vi "Autopatch-v2_mp285.vi"() -> ()   [LabVIEW 2018]
uses:
  <vilib>/vision/driver/NI_Vision_Acquisition_Software.lvlib
  <vilib>/DAQmx/create/channels.llb/DAQmx Create Channel (AO-Voltage-Basic).vi
  <vilib>/DAQmx/configure/timing.llb/DAQmx Timing (Sample Clock).vi
  <resource>/objmgr/daqmx.rc
  <vilib>/Analysis/NI_AALBase.lvlib
  <vilib>/Analysis/baseanly.llb/Mean (DBL).vi
  <vilib>/measure/NI_MABase.lvlib
  <vilib>/vision/NI_Vision_Development_Module.lvlib
  <vilib>/addons/control/pid/NI_PID_pid.lvlib
  <vilib>/addons/control/pid/pid.llb/PID (DBL).vi
  <vilib>/Analysis/NI_AALPro.lvlib
  <vilib>/DAQmx/write.llb/DAQmx Write (Analog DBL 1Chan 1Samp).vi
  <vilib>/DAQmx/configure/trigger.llb/DAQmx Start Trigger (Digital Edge).vi
  <vilib>/Waveform/WDTOps.llb/WDT Waveform Duration DBL.vi
  <vilib>/DAQmx/read.llb/DAQmx Read (Analog Wfm 1Chan NSamp).vi
  <vilib>/DAQmx/create/channels.llb/DAQmx Create Channel (AI-Voltage-Basic).vi
  <vilib>/DAQmx/write.llb/DAQmx Write (Analog Wfm 1Chan NSamp).vi
  <vilib>/userdefined/High Color/IMAQdx.ctl
panel:
  out "数据输出 2":string
  in  "模式（标准） 2":T1(ring)
  out "写入的字节 2":i32
  out "元素":string
  in  "自动对焦状态机":u16(ring) items=["自动对焦初始", "自动对焦循环", "自动对焦结束"]
  in  "自动扫描状态机":u16(ring) items=["自动扫描初始", "自动扫描循环", "自动扫描结束"]
  out "startY":dbl
  in  "手动暂停":bool
  out "Particle Measurements (Pixels)":dbl[][](array[numeric]) format="%.2f"
  in  "Pixel Measurements":T2[](array[typedef]) items=["Center of Mass X", "Center of Mass Y", "First Pixel X", "First Pixel Y", "Bounding Rect Left", "Bounding Rect Top", "Bounding Rect Right", "Bounding Rect Bottom", "Max Feret Diameter Start X", "Max Feret Diameter Start Y", "Max Feret Diameter End X", "Max Feret Diameter End Y", "Max Horiz. Segment Length Left", "Max Horiz. Segment Length Right", "Max Horiz. Segment Length Row", "-", "Bounding Rect Width", "Bounding Rect Height", "Bounding Rect Diagonal", "Perimeter", "Convex Hull Perimeter", "Holes' Perimeter", "Max Feret Diameter", "Equivalent Ellipse Major Axis", "Equivalent Ellipse Minor Axis", "Equivalent Ellipse Minor Axis (Feret)", "Equivalent Rect Long Side", "Equivalent Rect Short Side", "Equivalent Rect Diagonal", "Equivalent Rect Short Side (Feret)", "Average Horiz. Segment Length", "Average Vert. Segment Length", "Hydraulic Radius", "Waddel Disk Diameter", "-", "Area", "Holes' Area", "Particle & Holes' Area", "Convex Hull Area", "Image Area", "-", "Number of Holes", "Number of Horiz. Segments", "Number of Vert. Segments", "-", "Orientation", "Max Feret Diameter Orientation", "-", "% Area/Image Area", "% Area/(Particle & Holes' Area)", "Ratio of Equivalent Ellipse Axes", "Ratio of Equivalent Rect Sides", "-", "Elongation Factor", "Compactness Factor", "Heywood Circularity Factor", "Type Factor", "-", "Sum X", "Sum Y", "Sum XX", "Sum XY", "Sum YY", "Sum XXX", "Sum XXY", "Sum XYY", "Sum YYY", "-", "Moment of Inertia XX", "Moment of Inertia XY", "Moment of Inertia YY", "Moment of Inertia XXX", "Moment of Inertia XXY", "Moment of Inertia XYY", "Moment of Inertia YYY", "Norm. Moment of Inertia XX", "Norm. Moment of Inertia XY", "Norm. Moment of Inertia YY", "Norm. Moment of Inertia XXX", "Norm. Moment of Inertia XXY", "Norm. Moment of Inertia XYY", "Norm. Moment of Inertia YYY", "Hu Moment 1", "Hu Moment 2", "Hu Moment 3", "Hu Moment 4", "Hu Moment 5", "Hu Moment 6", "Hu Moment 7"]
  in  "手动换物镜":bool
  out "扫描变量":dbl=10.0
  in  "自动扫描":bool
  in  "自动移至工作位置":bool
  out "Z":dbl
  out "Y":dbl
  out "X":dbl
  in  "下降/向右 2":bool
  in  "下降步伐/um 2":dbl=1.0
  out "自动接触初始":i32
  in  "枚举":enum16{"200ms", "500ms", "1000ms", ""}(ring)
  out "dX/dt":dbl[](array[numeric])
  in  "下降/向右":bool
  in  "down":bool
  in  "up":bool
  out "Z轴坐标":string
  in  "调焦步伐/um":i64(ring)=3 items=["1", "10", "100", "1000", "10000"]
  in  "停止运动":bool
  in  "设置移动步长":bool
  in  "返回Z轴坐标":bool
  out "x*y":dbl
  out "电阻值":dbl
  in  "钳制电位":i16(ring) items=["0mv", "-70mv"]
  out "起始破膜时间":u32
  in  "自动破膜":bool
  in  "控制箱刺激ON\n/放大器刺激":bool=TRUE
  out "Image 2":T3(plugin-control)
  in  "对比图":bool
  in  "自动封接":bool
  in  "保存数据":bool
  out "是否匹配到？":bool
  in  "PID gains":T4={"proportional gain (Kc)"=-0.05, "integral time (Ti, min)"=0.0, "derivative time (Td, min)"=0.0} caption="PID增益" {"derivative time (Td, min)" format="%.3f"; "integral time (Ti, min)" format="%.3f"; "proportional gain (Kc)" format="%.3f"}
  in  "PID gains 2":T4={"proportional gain (Kc)"=0.05, "integral time (Ti, min)"=0.0, "derivative time (Td, min)"=0.0} caption="PID增益" {"derivative time (Td, min)" format="%.3f"; "integral time (Ti, min)" format="%.3f"; "proportional gain (Kc)" format="%.3f"}
  out "x+y 2":i16
  out "调焦值2":dbl
  out "调焦值3":dbl
  out "调焦值4":dbl
  out "对焦变量":dbl
  in  "聚焦值数组":dbl[](array[numeric])
  in  "下降步伐/um":dbl=1.0
  in  "自动接触":bool
  out "清晰度评价函数":dbl(graph)
  in  "针尖自动移动":bool
  in  "针尖细对焦":bool
  in  "针尖粗对焦":bool
  out "二值化":T3(plugin-control)
  in  "Range":cluster{"Lower value":sgl, "Upper value":sgl}={"Lower value"=0.0, "Upper value"=150.0} {"Upper value" format="%.2f"; "Lower value" format="%.2f"}
  in  "Operation":T5(ring)=enum."Dilate"
  in  "Number of Erosion":i32=10
  out "Particle Reports (Pixels)":T6(array[cluster]) {"Orientation" format="%.2f"; "Dimensions"."Height" format="%.2f"; "Dimensions"."Width" format="%.2f"; "Center of Mass"."Y" format="%.2f"; "Center of Mass"."X" format="%.2f"; "Bounding Rect"."Bottom" format="%.2f"; "Bounding Rect"."Right" format="%.2f"; "Bounding Rect"."Top" format="%.2f"; "Bounding Rect"."Left" format="%.2f"; "Number of Holes" format="%.2f"; "Area" format="%.2f"}
  out "Right":dbl
  out "目标坐标":i32[](array[numeric])
  in  "针尖模板匹配":bool=TRUE
  in  "基路径":path=path "E:/膜片/膜片钳/程序/CCD/模板40倍.jpg"
  out "Number of Matches":i32
  in  "Minimum Contrast":i32 min=0 max=255 step=1
  in  "Minimum Match Score":sgl=650.0 min=0 max=1000 format="%.2f"
  in  "Number of Matches Requested":i32=1 min=1
  out "Matches 2":T7(array[cluster]) {"Bounding Box"."y" format="%.2f"; "Bounding Box"."x" format="%.2f"; "Position"."y" format="%.2f"; "Position"."x" format="%.2f"; "Score" format="%.2f"; "Scale" format="%.2f"; "Angle" format="%.2f"}
  in  "Match Mode":u16(ring) items=["Shift Invariant", "Rotation Invariant"]
  out "针尖坐标":sgl[](array[numeric])
  in  "入液阻值校准":bool
  out "校准的入液阻值":dbl
  out "错误输出 3":errorcluster caption="错误输出"
  in  "低负开关":bool
  in  "低正开关":bool
  in  "大气压":bool
  in  "高负开关":bool
  in  "高正开关":bool
  in  "case":dbl
  out "测量值":dbl
  out "给定值":dbl
  out "输出气压波形图表":cluster{dbl, "低负":dbl}(graph)
  in  "低负":sgl(knob)=-0.45548448
  in  "高负":sgl(knob)=-5.0
  in  "低正":sgl(knob)=0.49642125 scale=0.0..2.0
  in  "高正":sgl(knob)=10.718505 scale=0.0..15.0
  in  "采样率":u32=255
  in  "DevIndex":i32
  in  "Holding Voltage":dbl=-70.0
  out "Negative Peak":dbl
  out "阻值波形图表":dbl(graph)
  out "Resistance(MΩ)":dbl
  out "！":bool
  in  "电压钳/电流钳":u16(ring) items=["Voltage Clamp", "Current Clamp"]
  out "电流信号波形图":waveform(dbl)(graph)
  in  "frequency":dbl=20.0
  in  "Averaging":i32=5
  in  "amplitude":dbl=0.01
  in  "阻值数组":dbl[](array[numeric])
  out "循环时间":u32
  out "Image":T3(plugin-control)
  out "错误输出":errorcluster
  in  "停止":bool
  in  "Session In":T8="cam1"
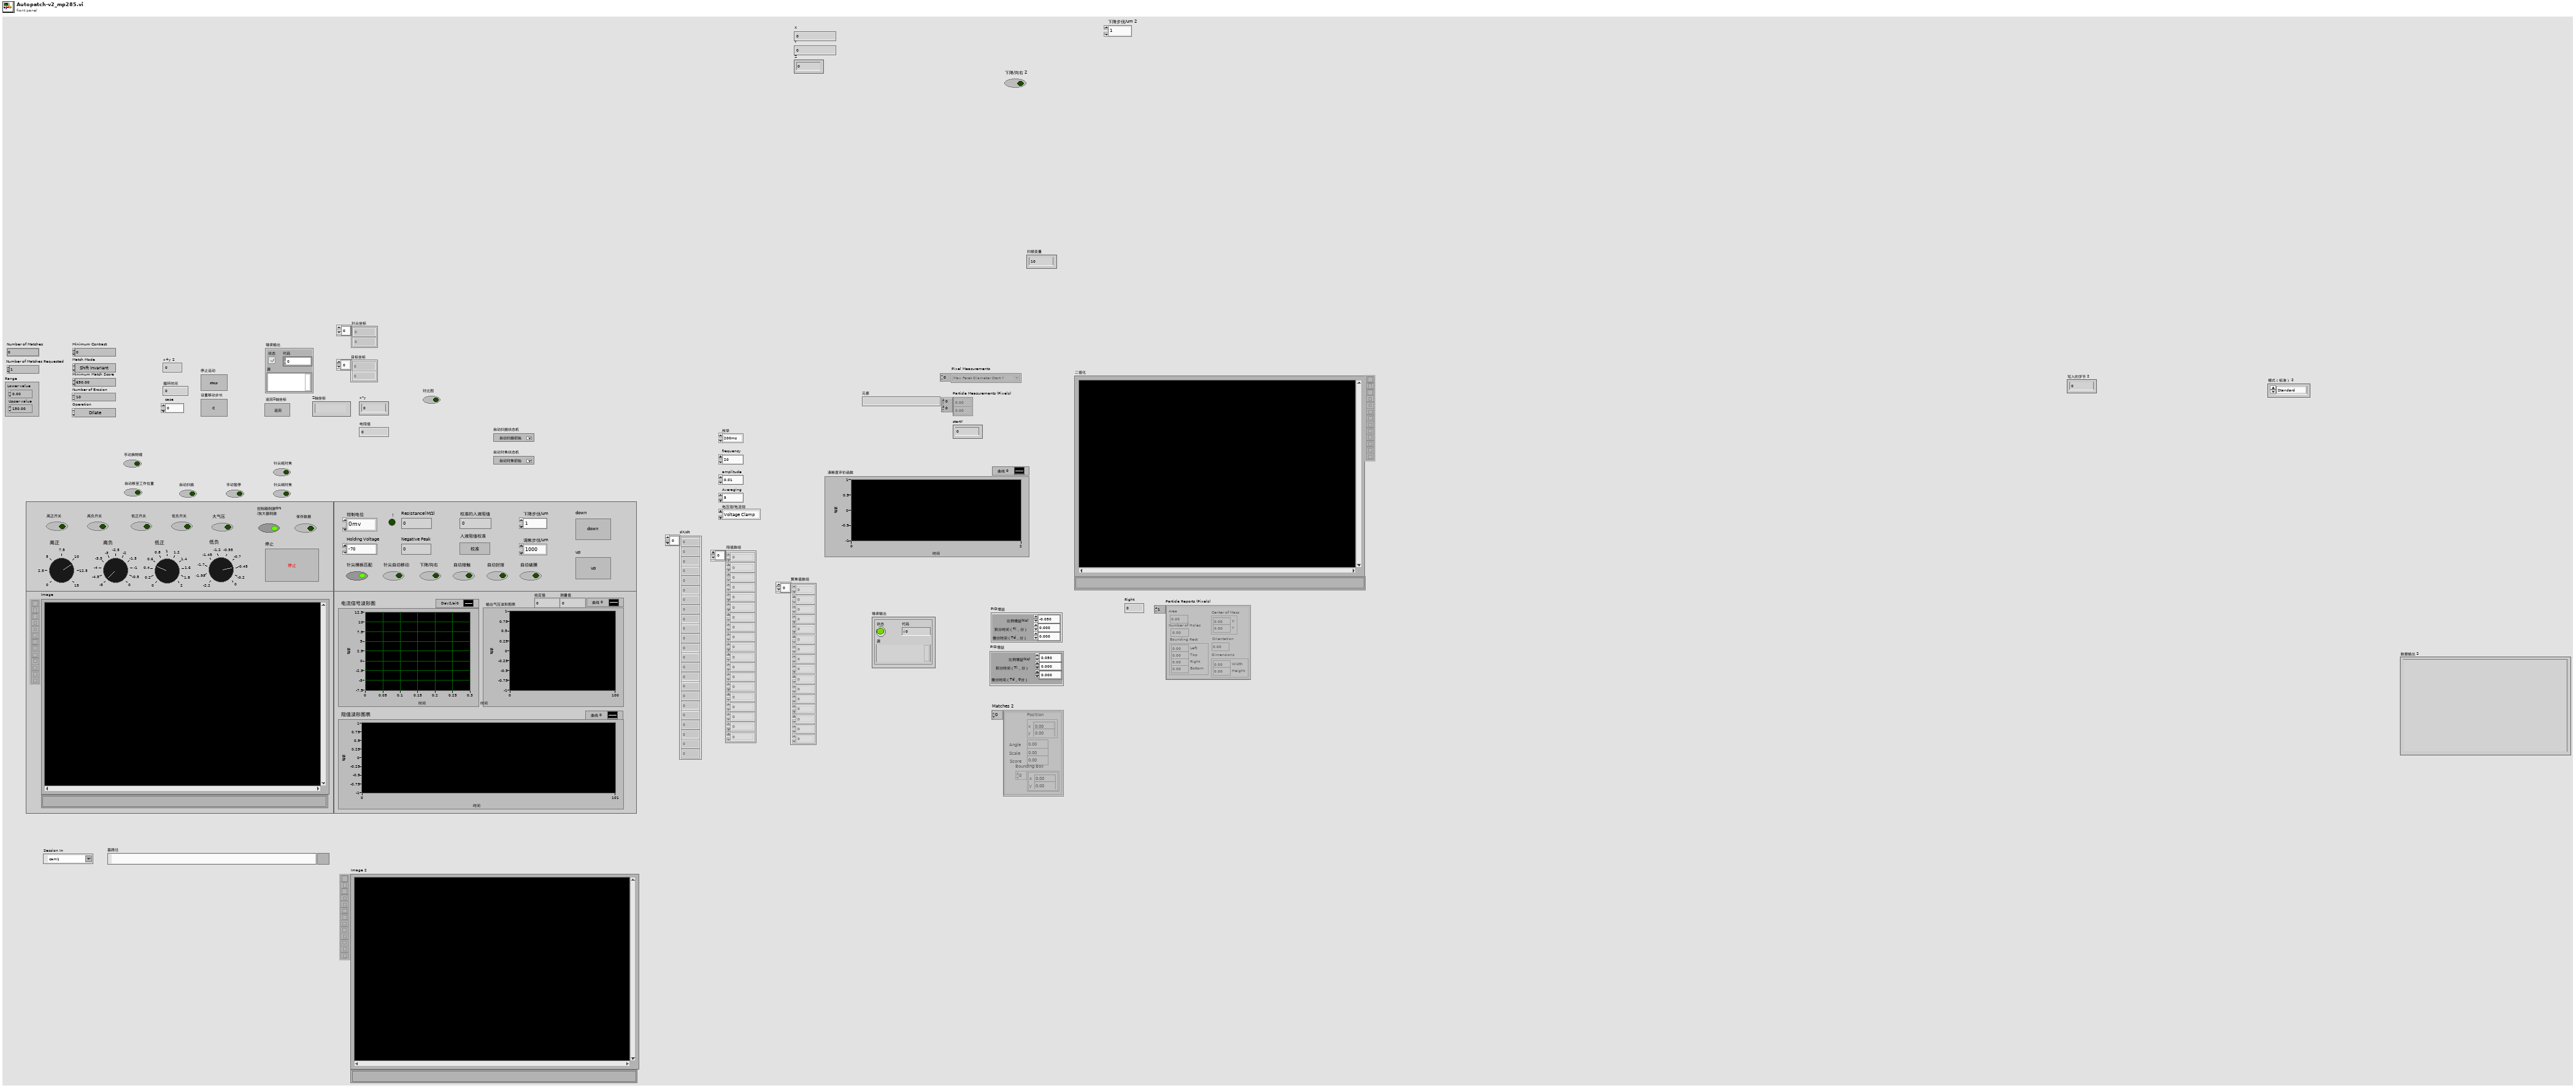
[diagram p1: front panel]
types:
  T1 = enum16{"Standard", "Buffered", "CRLF", "Immediate"}
  T2 = typedef "Particle Parameters" = i32
  T3 = typedef "IMAQ Image.ctl" = refnum<image>
  T4 = cluster{"proportional gain (Kc)":dbl, "integral time (Ti, min)":dbl, "derivative time (Td, min)":dbl}
  T5 = enum32{"AutoM", "Close", "Dilate", "Erode", "Gradient", "Gradient out", "Gradient in", "Hit miss", "Open", "PClose", "POpen", "Thick", "Thin"}
  T6 = cluster{"Area":dbl, "Number of Holes":dbl, "Bounding Rect":cluster{"Left":dbl, "Top":dbl, "Right":dbl, "Bottom":dbl}, "Center of Mass":cluster{"X":dbl, "Y":dbl}, "Orientation":dbl, "Dimensions":cluster{"Width":dbl, "Height":dbl}}[]
  T7 = cluster{"Position":cluster{"x":sgl, "y":sgl}, "Angle":sgl, "Scale":sgl, "Score":sgl, "Bounding Box":cluster{"x":sgl, "y":sgl}[]}[]
  T8 = typedef "IMAQdx.ctl" = refnum<k21>
  T9 = enum16{"open", "replace", "create", "open or create", "replace or create", "replace or create with confirmation"}
  T10 = typedef "Image Type" = u32
  T11 = cluster{"Averaging":i32, "frequency":dbl, "amplitude":dbl, "Proportion":dbl, "Fs":dbl}
  T12 = enum16{"Sine Wave", "Triangle Wave", "Square Wave", "Sawtooth Wave"}
  T13 = cluster{"Global Rectangle":i32[], "Contours":cluster{"Contour Type":u32, "ROI Type":u32, "Points":i32[]}[]}
  T14 = cluster{"Position":cluster{"x":sgl, "y":sgl}, "Angle":sgl, "Scale":sgl, "Score":sgl, "Bounding Box":cluster{"x":sgl, "y":sgl}[]}
  T15 = cluster{"Area":dbl, "Number of Holes":dbl, "Bounding Rect":cluster{"Left":dbl, "Top":dbl, "Right":dbl, "Bottom":dbl}, "Center of Mass":cluster{"X":dbl, "Y":dbl}, "Orientation":dbl, "Dimensions":cluster{"Width":dbl, "Height":dbl}}
  T16 = cluster{"Left":dbl, "Top":dbl, "Right":dbl, "Bottom":dbl}
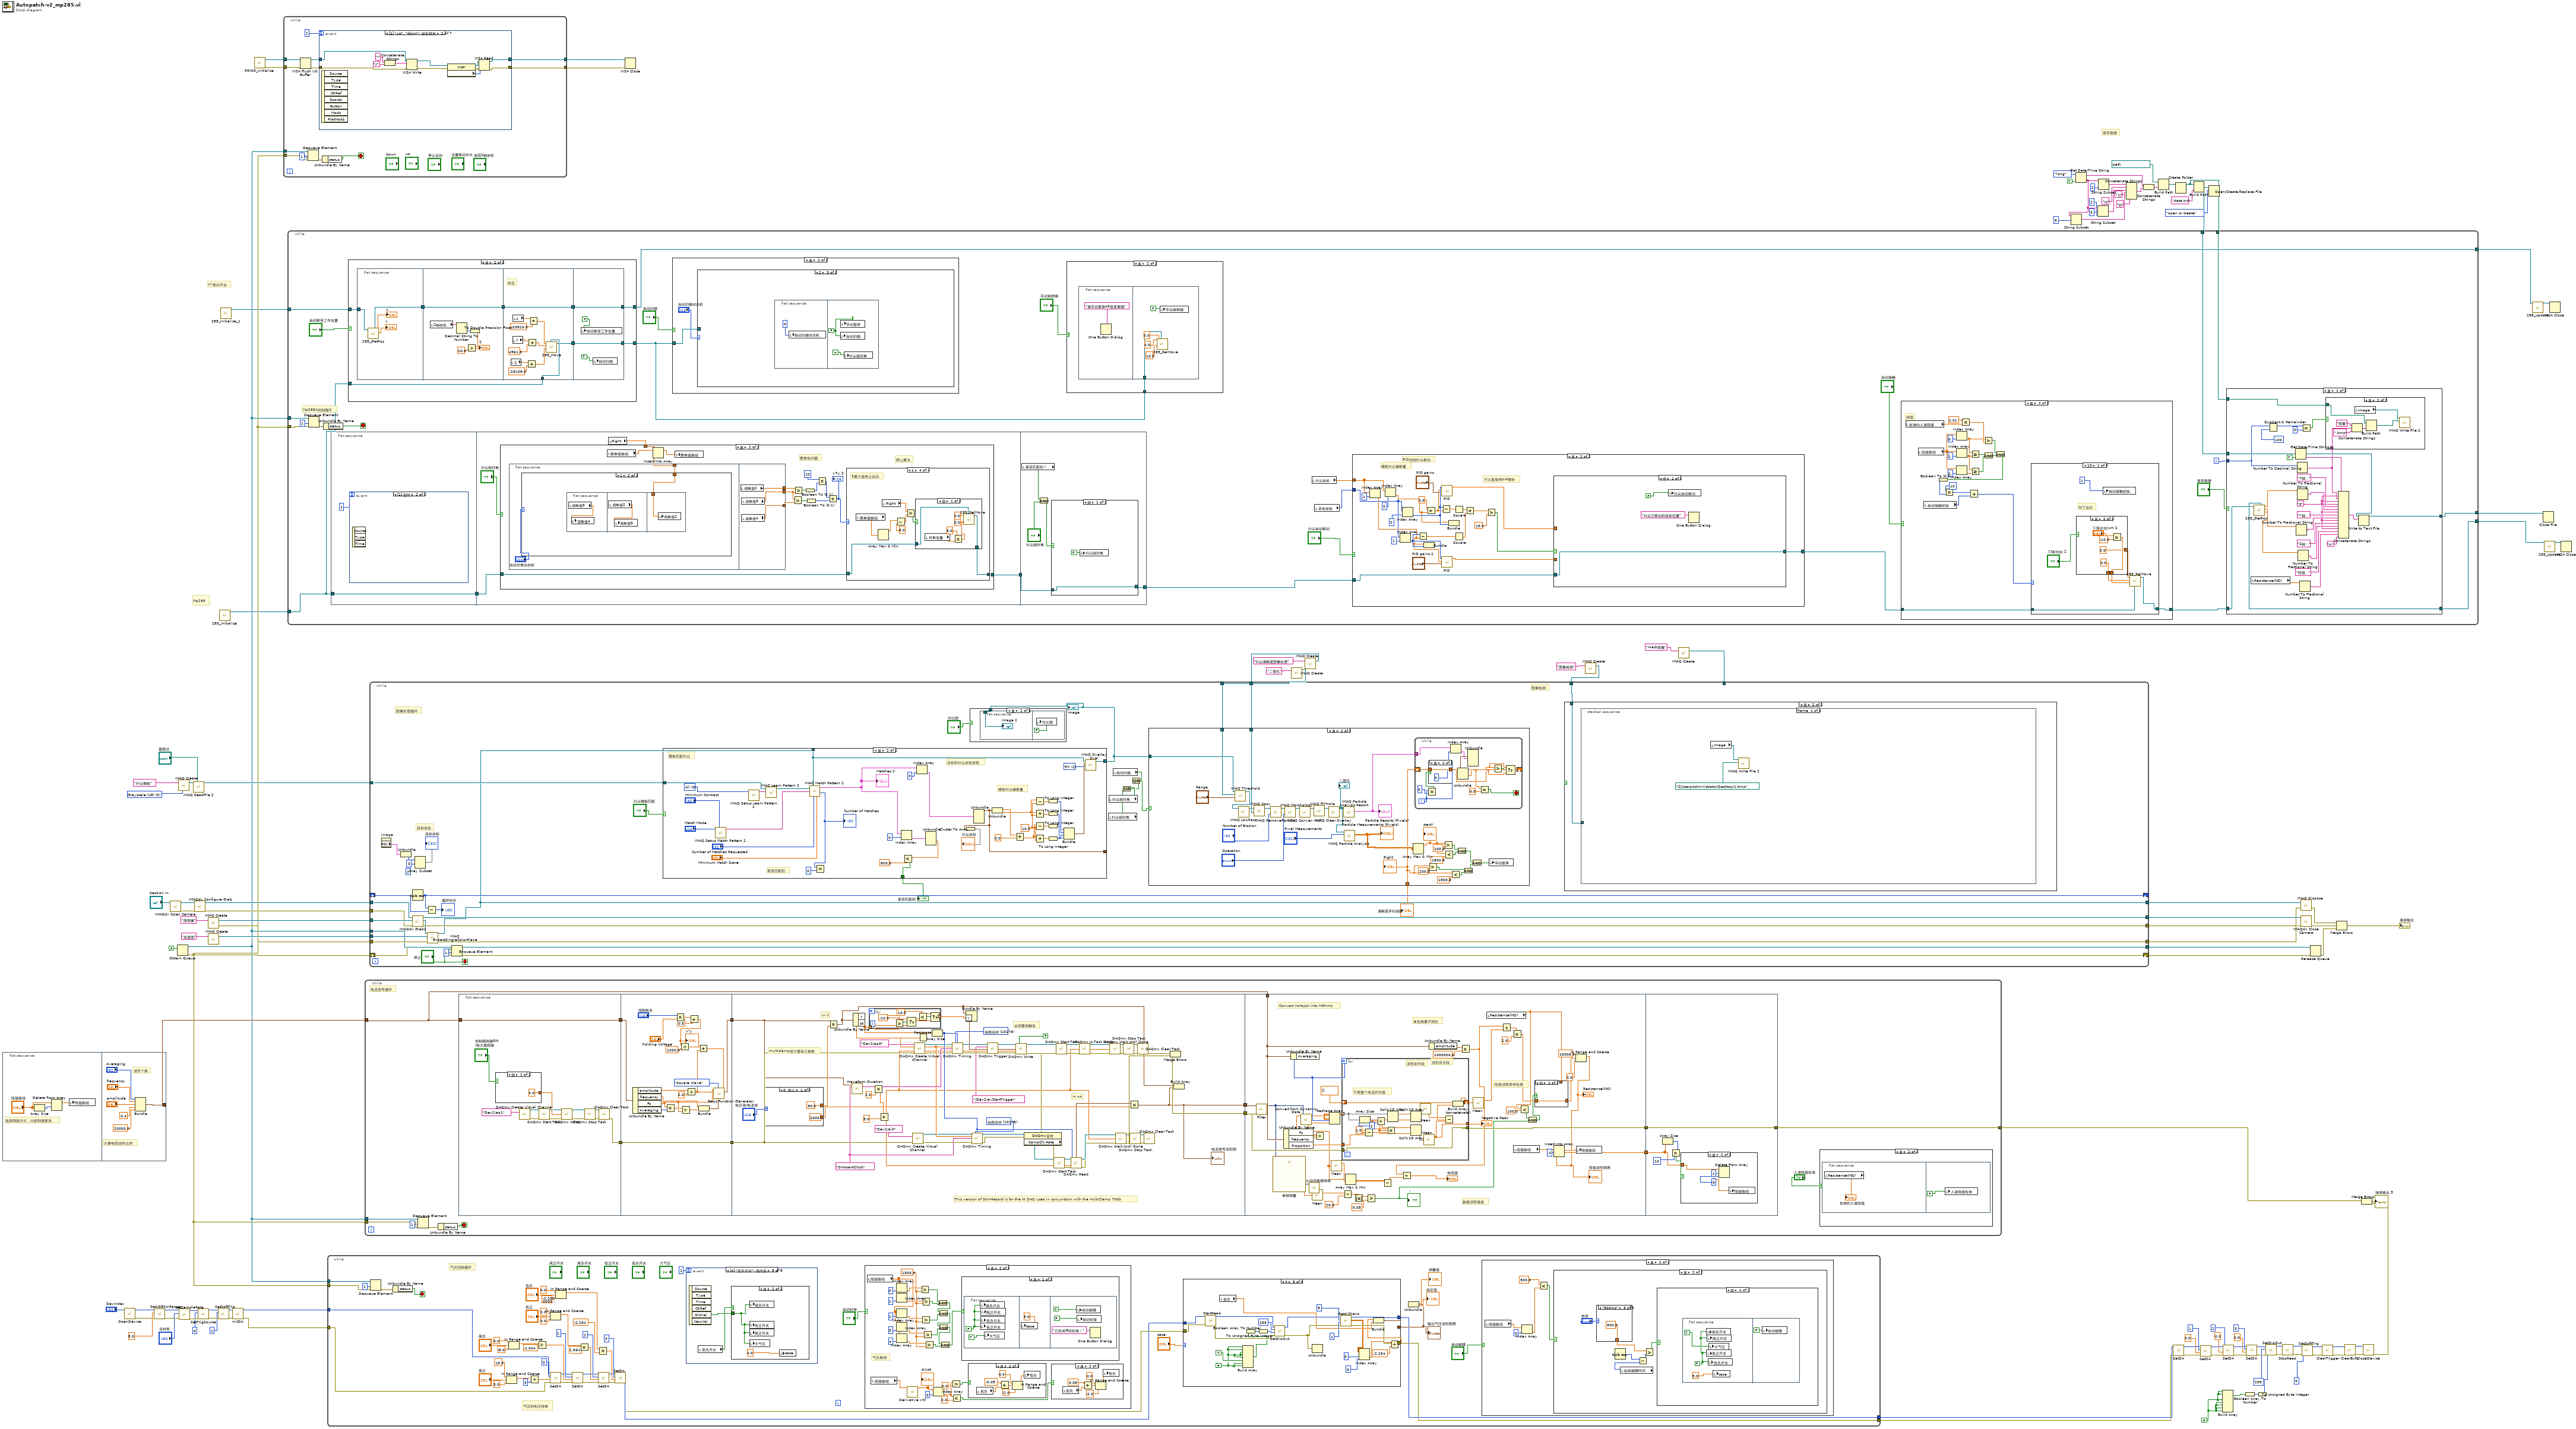
[diagram p0: block diagram]
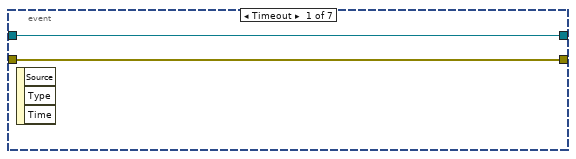
[diagram p2: hidden frame]
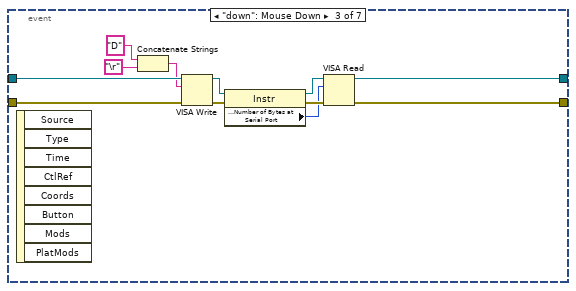
[diagram p3: hidden frame]
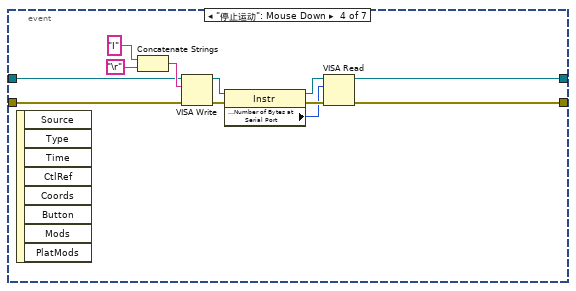
[diagram p4: hidden frame]
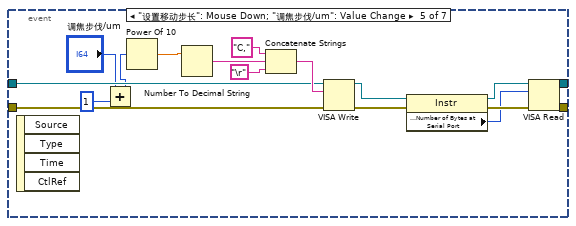
[diagram p5: hidden frame]
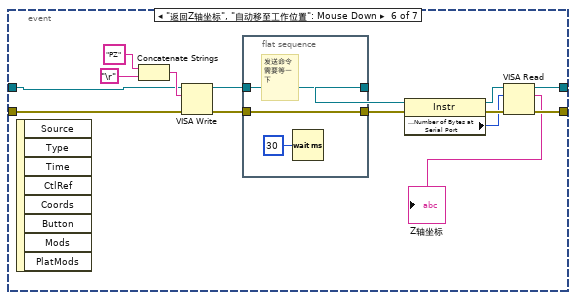
[diagram p6: hidden frame]
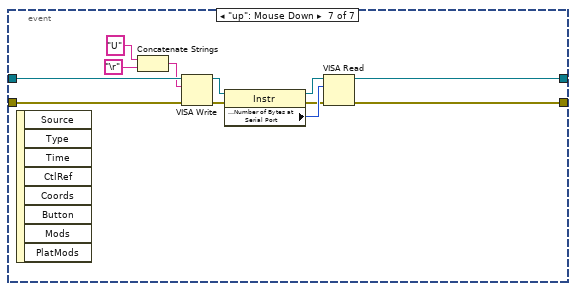
[diagram p7: hidden frame]
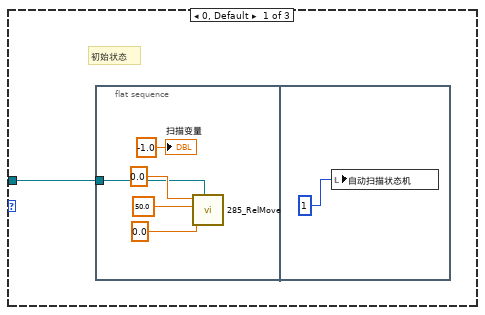
[diagram p10: hidden frame]
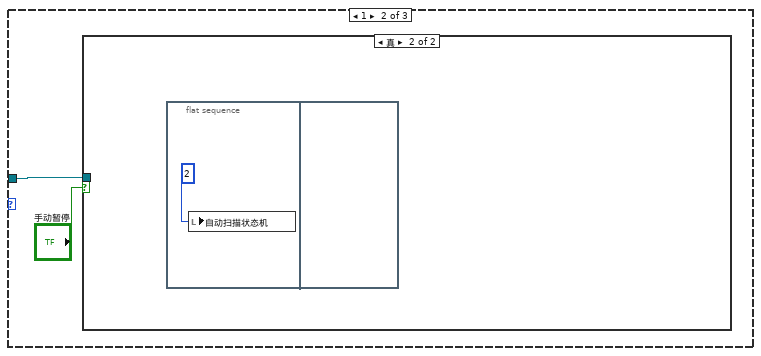
[diagram p11: hidden frame]
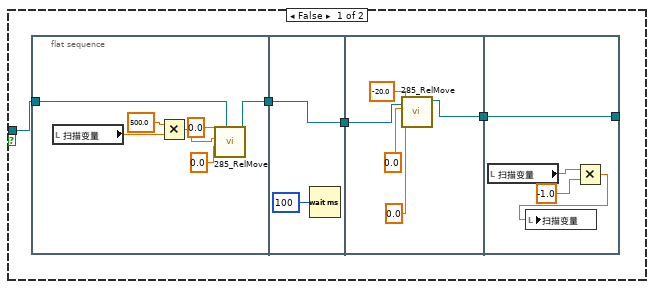
[diagram p12: hidden frame]
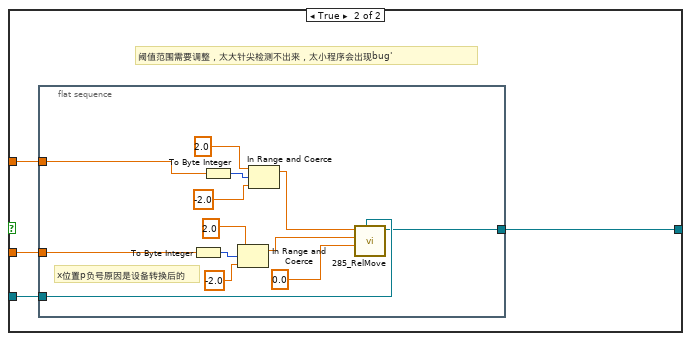
[diagram p17: hidden frame]
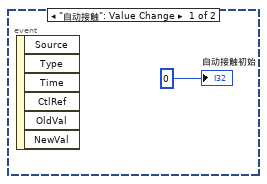
[diagram p18: hidden frame]
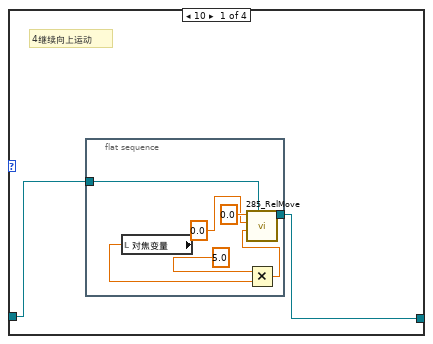
[diagram p20: hidden frame]
diagram:
  w50 = T10 0 items=["Grayscale (U8)", "Grayscale (I16)", "Grayscale (SGL)", "Complex (CSG)", "RGB (U32)", "HSL (U32)", "RGB (U64)", "Grayscale (U16)"] ("Image Type")
  w64 = FALSE
  # "XY移动平台"
  # "Mp285"
  # "保存数据"
  n1 = flat-sequence {
    tunnel: [w127] -> w111
    frame #0 {
      # "选择刺激方式，内部刺激更准"
      n2 = Array Size(array="阻值数组") -> (size(s)=w126:i32)
      n3 = Delete From Array(array="阻值数组", length=w126) -> (array with subset deleted=w124:dbl[])  [unwired: 1 in, 1 out]
      n4 = local write "阻值数组"(w124) -> ()
    }
    frame #1 {
      # "波形个数"
      # "计算电阻波形比例"
      n5 = Bundle("Averaging"="Averaging", "frequency"="frequency", "amplitude"="amplitude", "Proportion"=0.4, "Fs"=20000.0) -> (w127:T11)  [unwired: 1 in]
    }
  }
  n6 = call "OpenDevice.vi"("DevIndex"="DevIndex") -> ("错误输出"=w91:errorcluster, "DevIndex Output"=w89:i32)  [unwired: 9 in]
  n7 = call "SetUSB2AiRange.vi"("错误输入（无错误）"=w91, "Range"=sgl 5.0, "DevIndex"=w89) -> ("错误输出"=w100:errorcluster, "DevIndex Output"=w98:i32)  [unwired: 7 in]
  n8 = call <vilib>:"IMAQdx Open Camera.vi"("Session In"="Session In") -> ("error out"=w123:errorcluster, "Session Out"=w120:T8)  [unwired: 9 in]
  n9 = Obtain Queue(element data type=FALSE) -> (queue out=w8:refnum<queue>, error out=w7:errorcluster)  [unwired: 4 in, 1 out]
  n10 = call "IMAQ Create"("Image Name"="针尖模板", "Image Type"=w50) -> ("New Image"=w51:T3)  [unwired: 3 in, 1 out]
  n11 = call "SetSampleRate.vi"("错误输入（无错误）"=w100, "SampleRate"="采样率", "DevIndex"=w98) -> ("错误输出"=w101:errorcluster, "DevIndex Output"=w99:i32)  [unwired: 7 in]
  n12 = call "IMAQ ReadFile 2"("File Path"="基路径", "Image"=w51) -> ("Image Out"=w49:T3)  [unwired: 5 in, 4 out]
  n13 = call <vilib>:"IMAQdx Configure Grab.vi"("error in"=w123, "Session In"=w120) -> ("error out"=w108:errorcluster, "Session Out"=w121:T8)  [unwired: 8 in]
  n14 = call "SetTrigSource.vi"("错误输入（无错误）"=w101, "TrigSource"=u8 0, "DevIndex"=w99) -> ("错误输出"=w96:errorcluster, "DevIndex Output"=w95:i32)  [unwired: 7 in]
  n15 = call "IMAQ Create"("Image Name"="原图像") -> ("New Image"=w119:T3, "error out"=w106:errorcluster)  [unwired: 4 in]
  n16 = call "IMAQ Create"("Image Name"="灰度图") -> ("New Image"=w112:T3)  [unwired: 4 in, 1 out]
  n17 = call "SetSoftTrig.vi"("错误输入（无错误）"=w96, "Trig"=u8 1, "DevIndex"=w95) -> ("错误输出"=w92:errorcluster, "DevIndex Output"=w90:i32)  [unwired: 7 in]
  n18 = call "285_Initialize.vi"() -> ("VISA资源名称输出"=w6:refnum<visa-resource-name>)  [unwired: 10 in, 1 out]
  n19 = call "285_Initialize_1.vi"() -> ("VISA资源名称输出"=w5:refnum<visa-resource-name>)  [unwired: 10 in, 1 out]
  n20 = call "InitDA.vi"("错误输入（无错误）"=w92, "DevIndex"=w90) -> ("错误输出"=w86:errorcluster, "DevIndex Output"=w87:i32)  [unwired: 8 in]
  n21 = call "PRIOR_Initialize.vi"() -> ("错误输出"=w3:errorcluster, "VISA资源名称输出"=w4:refnum<visa-resource-name>)  [unwired: 10 in]
  n22 = while {
    tunnel: w4 -> [w142]
    tunnel: [w139] -> w9
    tunnel: [w143] -> w10
    tunnel: w8 -> [w136]
    tunnel: w7 -> [w135]
    tunnel: w3 -> [w133]
    stop <- w134 stop-if-true
    n23 = VISA Flush I/O Buffer(VISA resource name=w142, error in (no error)=w133) -> (VISA resource name out=w141:refnum<visa-resource-name>, error out=w140:errorcluster)  [unwired: 1 in]
    n24 = Dequeue Element(queue=w136, timeout in ms (-1)=1 ("超时毫秒(-1)"), error in (no error)=w135) -> (error out=w138:errorcluster)  [unwired: 3 out]
    n25 = event shown="[1] \"up\", \"down\": 鼠标释放" {
      selector: _ -> [_ _ _ _ _ _ _]
      dyn-events: _ -> [_ _ _ _ _ _ _]
      timeout: 1 -> [_ _ _ _ _ _ _]
      tunnel: [w146 w148 w170 w172 w190 w206 w229] -> w143
      tunnel: [w145 w147 w169 w171 w189 w205 w228] -> w139
      tunnel: w141 -> [w146 w150 w168 w174 w192 w208 w227]
      tunnel: w140 -> [w145 w149 w167 w173 w191 w207 w226]
      event Timeout {
        n26 = event-data() -> ()  [unwired: 1 in, 3 out]
      }
      event "up", "down": Mouse Up {
        n27 = event-data() -> ()  [unwired: 1 in, 8 out]
        n28 = Concatenate Strings("I" ("写入缓冲区"), "\r") -> (w158:string)
        n29 = VISA Write ("VISA写入")(VISA resource name=w150, write buffer=w158, error in (no error)=w149) -> (VISA resource name out=w152:refnum<visa-resource-name>, error out=w151:errorcluster)  [unwired: 1 out]
        n30 = property class="Instr"(reference=w152, error in=w151) -> (reference out=w153:refnum<visa-resource-name>, error out=w154:errorcluster, "Serial Settings:Number of Bytes at Serial Port"=w155:u32)
        n31 = VISA Read(VISA resource name=w153, byte count=w155, error in (no error)=w154) -> (VISA resource name out=w148:refnum<visa-resource-name>, error out=w147:errorcluster)  [unwired: 2 out]
      }
      event "down": Mouse Down {
        n32 = event-data() -> ()  [unwired: 1 in, 8 out]
        n33 = Concatenate Strings("D" ("写入缓冲区"), "\r") -> (w159:string)
        n34 = VISA Write ("VISA写入")(VISA resource name=w168, write buffer=w159, error in (no error)=w167) -> (VISA resource name out=w165:refnum<visa-resource-name>, error out=w166:errorcluster)  [unwired: 1 out]
        n35 = property class="Instr"(reference=w165, error in=w166) -> (reference out=w164:refnum<visa-resource-name>, error out=w163:errorcluster, "Serial Settings:Number of Bytes at Serial Port"=w162:u32)
        n36 = VISA Read(VISA resource name=w164, byte count=w162, error in (no error)=w163) -> (VISA resource name out=w170:refnum<visa-resource-name>, error out=w169:errorcluster)  [unwired: 2 out]
      }
      event "停止运动": Mouse Down {
        n37 = event-data() -> ()  [unwired: 1 in, 8 out]
        n38 = Concatenate Strings("I" ("写入缓冲区"), "\r") -> (w175:string)
        n39 = VISA Write ("VISA写入")(VISA resource name=w174, write buffer=w175, error in (no error)=w173) -> (VISA resource name out=w181:refnum<visa-resource-name>, error out=w182:errorcluster)  [unwired: 1 out]
        n40 = property class="Instr"(reference=w181, error in=w182) -> (reference out=w180:refnum<visa-resource-name>, error out=w179:errorcluster, "Serial Settings:Number of Bytes at Serial Port"=w178:u32)
        n41 = VISA Read(VISA resource name=w180, byte count=w178, error in (no error)=w179) -> (VISA resource name out=w172:refnum<visa-resource-name>, error out=w171:errorcluster)  [unwired: 2 out]
      }
      event "设置移动步长": Mouse Down; "调焦步伐/um": Value Change {
        n42 = event-data() -> ()  [unwired: 1 in, 4 out]
        n43 = Add(x="调焦步伐/um", y=i64 1) -> (x+y=w183:i64)
        n44 = Power Of 10(x=w183) -> (10^x=w186:dbl)
        n45 = Number To Decimal String(number=w186) -> (decimal integer string=w187:string)  [unwired: 1 in]
        n46 = Concatenate Strings("C," ("写入缓冲区"), w187, "\r") -> (w193:string)
        n47 = VISA Write ("VISA写入")(VISA resource name=w192, write buffer=w193, error in (no error)=w191) -> (VISA resource name out=w198:refnum<visa-resource-name>, error out=w199:errorcluster)  [unwired: 1 out]
        n48 = property class="Instr"(reference=w198, error in=w199) -> (reference out=w197:refnum<visa-resource-name>, error out=w196:errorcluster, "Serial Settings:Number of Bytes at Serial Port"=w195:u32)
        n49 = VISA Read(VISA resource name=w197, byte count=w195, error in (no error)=w196) -> (VISA resource name out=w190:refnum<visa-resource-name>, error out=w189:errorcluster)  [unwired: 2 out]
      }
      event "返回Z轴坐标", "自动移至工作位置": Mouse Down {
        n50 = event-data() -> ()  [unwired: 1 in, 8 out]
        n51 = Concatenate Strings("PZ" ("写入缓冲区"), "\r") -> (w210:string)
        n52 = VISA Write ("VISA写入")(VISA resource name=w208, write buffer=w210, error in (no error)=w207) -> (VISA resource name out=w204:refnum<visa-resource-name>, error out=w203:errorcluster)  [unwired: 1 out]
        n53 = flat-sequence {
          tunnel: w204 -> [w216]
          tunnel: w203 -> [w217]
          tunnel: [w217] -> w201
          tunnel: [w216] -> w202
          frame #0 {
            # "发送命令需要等一下"
            n54 = Wait (ms)(milliseconds to wait=u32 30 ("等待时间（毫秒）")) -> ()  [unwired: 1 out]
          }
        }
        n55 = property class="Instr"(reference=w202, error in=w201) -> (reference out=w214:refnum<visa-resource-name>, error out=w213:errorcluster, "Serial Settings:Number of Bytes at Serial Port"=w212:u32)
        n56 = VISA Read(VISA resource name=w214, byte count=w212, error in (no error)=w213) -> (VISA resource name out=w206:refnum<visa-resource-name>, read buffer=→"Z轴坐标":string, error out=w205:errorcluster)  [unwired: 1 out]
      }
      event "up": Mouse Down {
        n57 = event-data() -> ()  [unwired: 1 in, 8 out]
        n58 = Concatenate Strings("U" ("写入缓冲区"), "\r") -> (w223:string)
        n59 = VISA Write ("VISA写入")(VISA resource name=w227, write buffer=w223, error in (no error)=w226) -> (VISA resource name out=w222:refnum<visa-resource-name>, error out=w221:errorcluster)  [unwired: 1 out]
        n60 = property class="Instr"(reference=w222, error in=w221) -> (reference out=w219:refnum<visa-resource-name>, error out=w218:errorcluster, "Serial Settings:Number of Bytes at Serial Port"=w220:u32)
        n61 = VISA Read(VISA resource name=w219, byte count=w220, error in (no error)=w218) -> (VISA resource name out=w229:refnum<visa-resource-name>, error out=w228:errorcluster)  [unwired: 2 out]
      }
    }
    n62 = Unbundle By Name(w138) -> ("status"=w134:bool)
  }
  n63 = while {
    tunnel: w87 -> [w242]
    tunnel: w8 -> [w281]
    tunnel: w7 -> [w280]
    tunnel: [w234] -> w12
    tunnel: w86 -> [w241]
    tunnel: [w232] -> w11
    stop <- w277 stop-if-true
    # "气压控制循环"
    # "气压到电压转换"
    n64 = Dequeue Element(queue=w281, timeout in ms (-1)=1 ("超时毫秒(-1)"), error in (no error)=w280) -> (error out=w278:errorcluster)  [unwired: 3 out]
    n65 = Unbundle By Name(w278) -> ("status"=w277:bool)
    n66 = In Range and Coerce(upper limit=sgl 15.0 ("上限"), x="高正", lower limit=sgl 0.0 ("下限")) -> (coerced(x)=w245:sgl)  [unwired: 1 out]
    n67 = In Range and Coerce(upper limit=sgl 0.0 ("上限"), x="高负", lower limit=sgl -5.0 ("下限")) -> (coerced(x)=w249:sgl)  [unwired: 1 out]
    n68 = Divide(x=w245, y=3) -> (x/y=w266:sgl)
    n69 = Divide(x=w249, y=-1.004) -> (x/y=w262:dbl)
    n70 = In Range and Coerce(upper limit=sgl 2.0 ("上限"), x="低正", lower limit=sgl 0.0 ("下限")) -> (coerced(x)=w253:sgl)  [unwired: 1 out]
    n71 = call "SetDA.vi"("错误输入（无错误）"=w241, "DAVolt"=w266, "DANum"=u8 0, "DevIndex"=w242) -> ("错误输出"=w275:errorcluster, "DevIndex Output"=w276:i32)  [unwired: 6 in]
    n72 = In Range and Coerce(upper limit=sgl 0.0 ("上限"), x="低负", lower limit=sgl -2.2 ("下限")) -> (coerced(x)=w255:sgl)  [unwired: 1 out]
    n73 = call "SetDA.vi"("错误输入（无错误）"=w275, "DAVolt"=w262, "DANum"=u8 1, "DevIndex"=w276) -> ("错误输出"=w274:errorcluster, "DevIndex Output"=w273:i32)  [unwired: 6 in]
    n74 = Multiply(x=w253, y=2.564) -> (x*y=w259:dbl)
    n75 = Multiply(x=w255, y=-2.294) -> (x*y=w260:dbl)
    n76 = call "SetDA.vi"("错误输入（无错误）"=w274, "DAVolt"=w259, "DANum"=u8 2, "DevIndex"=w273) -> ("错误输出"=w271:errorcluster, "DevIndex Output"=w272:i32)  [unwired: 6 in]
    n77 = call "SetDA.vi"("错误输入（无错误）"=w271, "DAVolt"=w260, "DANum"=u8 3, "DevIndex"=w272) -> ("错误输出"=w235:errorcluster, "DevIndex Output"=w236:i32)  [unwired: 6 in]
    n78 = event shown="[4] \"低负开关\": 值改变" {
      selector: _ -> [_ _ _ _ _ _ _ _]
      dyn-events: _ -> [_ _ _ _ _ _ _ _]
      timeout: 1 -> [_ _ _ _ _ _ _ _]
      event "高正开关": Value Change {
        n79 = event-data() -> ("OldVal"=w355:bool)  [unwired: 1 in, 5 out]
        n80 = local read "高正开关"() -> (w356:bool)
        n81 = case shown="真" w356 {
          tunnel: w355 -> [_ w358]
          frame False {
          }
          frame True {
            n82 = local write "高负开关"(w358) -> ()
            n83 = local write "低负开关"(w358) -> ()
            n84 = local write "低正开关"(w358) -> ()
            n85 = local write "大气压"(w358) -> ()
            n86 = local write "case"(1.0) -> ()
          }
        }
      }
      event Timeout {
        n87 = event-data() -> ()  [unwired: 1 in, 3 out]
      }
      event "大气压": Value Change {
        n88 = event-data() -> ("OldVal"=w359:bool)  [unwired: 1 in, 5 out]
        n89 = local read "大气压"() -> (w360:bool)
        n90 = case shown="真" w360 {
          tunnel: w359 -> [_ w362]
          frame False {
          }
          frame True {
            n91 = local write "高负开关"(w362) -> ()
            n92 = local write "低正开关"(w362) -> ()
            n93 = local write "低负开关"(w362) -> ()
            n94 = local write "高正开关"(w362) -> ()
            n95 = local write "case"(5.0) -> ()
          }
        }
      }
      event "低正开关": Value Change {
        n96 = event-data() -> ("OldVal"=w364:bool)  [unwired: 1 in, 5 out]
        n97 = local read "低正开关"() -> (w363:bool)
        n98 = case shown="真" w363 {
          tunnel: w364 -> [_ w366]
          frame False {
          }
          frame True {
            n99 = local write "高正开关"(w366) -> ()
            n100 = local write "高负开关"(w366) -> ()
            n101 = local write "低负开关"(w366) -> ()
            n102 = local write "大气压"(w366) -> ()
            n103 = local write "case"(3.0) -> ()
          }
        }
      }
      event "低负开关": Value Change {
        n104 = event-data() -> ("OldVal"=w368:bool)  [unwired: 1 in, 5 out]
        n105 = local read "低负开关"() -> (w367:bool)
        n106 = case shown="真" w367 {
          tunnel: w368 -> [_ w370]
          frame False {
          }
          frame True {
            n107 = local write "高负开关"(w370) -> ()
            n108 = local write "低正开关"(w370) -> ()
            n109 = local write "高正开关"(w370) -> ()
            n110 = local write "大气压"(w370) -> ()
            n111 = local write "case"(4.0) -> ()
          }
        }
      }
      event "高负开关": Value Change {
        n112 = event-data() -> ("OldVal"=w372:bool)  [unwired: 1 in, 5 out]
        n113 = local read "高负开关"() -> (w371:bool)
        n114 = case shown="真" w371 {
          tunnel: w372 -> [_ w374]
          frame False {
          }
          frame True {
            n115 = local write "低正开关"(w374) -> ()
            n116 = local write "低负开关"(w374) -> ()
            n117 = local write "高正开关"(w374) -> ()
            n118 = local write "大气压"(w374) -> ()
            n119 = local write "case"(2.0) -> ()
          }
        }
      }
      event "自动封接": Value Change {
        # "初始值"
        n120 = event-data() -> ()  [unwired: 1 in, 6 out]
        n121 = local write "低负"(-0.66) -> ()
      }
      event "自动破膜": Value Change {
        n122 = event-data() -> ()  [unwired: 1 in, 6 out]
        n123 = Tick Count (ms)() -> (millisecond timer value=→"起始破膜时间":u32)
      }
    }
    n124 = case shown="真" "自动封接" {
      frame False {
      }
      frame True {
        w317 = 1300.0 ("y")
        # "气压微调"
        n125 = local read "阻值数组"() -> (w318:dbl[])
        n126 = local read "阻值数组"() -> (w312:dbl[])
        n127 = Index Array(array=w318, index=0 ("索引")) -> (element=w320:dbl)
        n128 = Index Array(array=w318, index=1 ("索引")) -> (element=w319:dbl)
        n129 = Index Array(array=w318, index=2 ("索引")) -> (element=w328:dbl)
        n130 = Index Array(array=w318, index=3 ("索引")) -> (element=w327:dbl)
        n131 = Index Array(array=w318, index=4 ("索引")) -> (element=w326:dbl)
        n132 = call <vilib>:"Derivative x(t).vi"("X"=w312) -> ("dX/dt"=w309:dbl[])  [unwired: 9 in, 1 out]
        "dX/dt" <- w309
        n133 = Greater?(x=w320, y=w317) -> (0:w325:bool)
        n134 = Greater?(x=w328, y=w317) -> (0:w323:bool)
        n135 = Greater?(x=w319, y=w317) -> (0:w324:bool)
        n136 = Greater?(x=w327, y=w317) -> (0:w322:bool)
        n137 = Greater?(x=w326, y=w317) -> (0:w321:bool)
        n138 = Index Array(array=w309, index=0 ("索引")) -> (element=w305:dbl)
        n139 = And(x=w325, y=w324) -> (x .and. y?=w316:bool)
        n140 = And(x=w316, y=w323) -> (x .and. y?=w315:bool)
        n141 = And(x=w315, y=w322) -> (x .and. y?=w314:bool)
        n142 = And(x=w314, y=w321) -> (x .and. y?=w313:bool)
        n143 = Greater?(x=w305, y=0.0) -> (0:w311:bool)
        n144 = Less?(x=w305, y=0.0) -> (x < y?=w310:bool)
        n145 = case shown="真" w313 {
          frame True {
            n146 = flat-sequence {
              frame #0 {
                w346 = FALSE
                n147 = local write "高负开关"(w346) -> ()
                n148 = local write "低负开关"(w346) -> ()
                n149 = local write "低正开关"(w346) -> ()
                n150 = local write "高正开关"(w346) -> ()
                n151 = local write "大气压"(TRUE) -> ()
              }
              frame #1 {
                n152 = local write "case"(5.0) -> ()
              }
              frame #2 {
                n153 = local write "自动破膜"(TRUE) -> ()
                n154 = local write "自动封接"(FALSE) -> ()
                n155 = One Button Dialog(message="已形成G欧封接！" ("消息")) -> ()  [unwired: 1 in, 1 out]
              }
            }
          }
          frame False {
            n156 = flat-sequence {
              frame #0 {
                w352 = FALSE
                n157 = local write "高负开关"(w352) -> ()
                n158 = local write "低正开关"(w352) -> ()
                n159 = local write "高正开关"(w352) -> ()
                n160 = local write "低负开关"(TRUE) -> ()
                n161 = local write "大气压"(w352) -> ()
              }
              frame #1 {
                n162 = local write "case"(4.0) -> ()
              }
            }
          }
        }
        n163 = case shown="真" w311 {
          frame False {
          }
          frame True {
            n164 = local read "低负"() -> (w341:sgl)
            n165 = Add(x=-0.05, y=w341) -> (x+y=w344:dbl)
            n166 = In Range and Coerce(upper limit=0.0, x=w344, lower limit=-2.0) -> (coerced(x)=w340:dbl)  [unwired: 1 out]
            n167 = local write "低负"(w340) -> ()
          }
        }
        n168 = case shown="真" w310 {
          frame False {
          }
          frame True {
            n169 = local read "低负"() -> (w335:sgl)
            n170 = Add(x=0.05, y=w335) -> (x+y=w338:dbl)
            n171 = In Range and Coerce(upper limit=0.0, x=w338, lower limit=-2.0) -> (coerced(x)=w334:dbl)  [unwired: 1 out]
            n172 = local write "低负"(w334) -> ()
          }
        }
      }
    }
    n173 = case shown="4" "case" {
      tunnel: w236 -> [w380 w400 w422 w446 w470 w483]
      tunnel: w235 -> [w379 w399 w421 w445 w469 w482]
      tunnel: [w380 w382 w413 w440 w462 w480] -> w234
      tunnel: [w379 w390 w414 w439 w463 w479] -> w232
      tunnel: [w377 w381 w405 w429 w453 w477] -> w238
      frame Default {
        w378 = 0.0
        n174 = Bundle(w378, w378) -> (w377:cluster{dbl, dbl})  [unwired: 1 in]
      }
      frame 1 {
        w397 = TRUE
        w398 = FALSE
        n175 = Build Array(w398, w397, w397, w398, w398, w398, w398, w398) -> (w401:bool[])
        n176 = Boolean Array To Number(Boolean array=w401) -> (number=w404:u32)
        n177 = To Unsigned Byte Integer(number=w404) -> (unsigned 8bit integer=w403:u8)
        n178 = call "StartRead.vi"("错误输入（无错误）"=w399, "DevIndex"=w400) -> ("错误输出"=w395:errorcluster, "DevIndex Output"=w396:i32)  [unwired: 8 in]
        n179 = call "SetDioOut.vi"("错误输入（无错误）"=w395, "DioOut"=w403, "DioChanSel"=u8 255, "DevIndex"=w396) -> ("错误输出"=w391:errorcluster, "DevIndex Output"=w392:i32)  [unwired: 6 in]
        n180 = call "GetAiChans.vi"("错误输入（无错误）"=w391, "Num"=u32 1, "ChanSel"=u16 1, "DevIndex"=w392) -> ("错误输出"=w390:errorcluster, "Ai"=w387:sgl[][], "DevIndex Output"=w382:i32)  [unwired: 4 in, 1 out]
        n181 = Index Array(array=w387, index (row)=0, index (col)=0) -> (element=w384:sgl)
        n182 = local read "高正"() -> (w386:sgl)
        n183 = Multiply(x=w384, y=3) -> (x*y=w383:sgl)
        n184 = Bundle(w383, "高正"=w386) -> (w381:cluster{sgl, "高正":sgl})  [unwired: 1 in]
      }
      frame 2 {
        w420 = TRUE
        w419 = FALSE
        n185 = Build Array(w419, w420, w419, w419, w420, w419, w419, w419) -> (w423:bool[])
        n186 = Boolean Array To Number(Boolean array=w423) -> (number=w428:u32)
        n187 = To Unsigned Byte Integer(number=w428) -> (unsigned 8bit integer=w427:u8)
        n188 = call "StartRead.vi"("错误输入（无错误）"=w421, "DevIndex"=w422) -> ("错误输出"=w424:errorcluster, "DevIndex Output"=w425:i32)  [unwired: 8 in]
        n189 = call "SetDioOut.vi"("错误输入（无错误）"=w424, "DioOut"=w427, "DioChanSel"=u8 255, "DevIndex"=w425) -> ("错误输出"=w415:errorcluster, "DevIndex Output"=w416:i32)  [unwired: 6 in]
        n190 = call "GetAiChans.vi"("错误输入（无错误）"=w415, "Num"=u32 1, "ChanSel"=u16 2, "DevIndex"=w416) -> ("错误输出"=w414:errorcluster, "Ai"=w410:sgl[][], "DevIndex Output"=w413:i32)  [unwired: 4 in, 1 out]
        n191 = Unbundle(w415) -> ()  [unwired: 3 out]
        n192 = Index Array(array=w410, index (row)=0, index (col)=0) -> (element=w408:sgl)
        n193 = local read "高负"() -> (w409:sgl)
        n194 = Multiply(x=w408, y=-1.004) -> (x*y=w406:dbl)
        n195 = Bundle(w406, "高负"=w409) -> (w405:cluster{dbl, "高负":sgl})  [unwired: 1 in]
      }
      frame 3 {
        w431 = FALSE
        n196 = Build Array(w431, w431, w431, TRUE, w431, w431, w431, w431) -> (w447:bool[])
        n197 = Boolean Array To Number(Boolean array=w447) -> (number=w452:u32)
        n198 = To Unsigned Byte Integer(number=w452) -> (unsigned 8bit integer=w451:u8)
        n199 = call "StartRead.vi"("错误输入（无错误）"=w445, "DevIndex"=w446) -> ("错误输出"=w448:errorcluster, "DevIndex Output"=w449:i32)  [unwired: 8 in]
        n200 = call "SetDioOut.vi"("错误输入（无错误）"=w448, "DioOut"=w451, "DioChanSel"=u8 255, "DevIndex"=w449) -> ("错误输出"=w441:errorcluster, "DevIndex Output"=w442:i32)  [unwired: 6 in]
        n201 = call "GetAiChans.vi"("错误输入（无错误）"=w441, "Num"=u32 1, "ChanSel"=u16 4, "DevIndex"=w442) -> ("错误输出"=w439:errorcluster, "Ai"=w436:sgl[][], "DevIndex Output"=w440:i32)  [unwired: 4 in, 1 out]
        n202 = Unbundle(w441) -> ()  [unwired: 3 out]
        n203 = Index Array(array=w436, index (row)=0, index (col)=0) -> (element=w434:sgl)
        n204 = local read "低正"() -> (w435:sgl)
        n205 = Divide(x=w434, y=2.564) -> (x/y=w432:dbl)
        n206 = Bundle(w432, "低正"=w435) -> (w429:cluster{dbl, "低正":sgl})  [unwired: 1 in]
      }
      frame 4 {
        w454 = FALSE
        n207 = call "StartRead.vi"("错误输入（无错误）"=w469, "DevIndex"=w470) -> ("错误输出"=w472:errorcluster, "DevIndex Output"=w473:i32)  [unwired: 8 in]
        n208 = local read "低负"() -> (w458:sgl)
        n209 = Build Array(w454, w454, w454, w454, w454, TRUE, w454, w454) -> (w471:bool[])
        n210 = Boolean Array To Number(Boolean array=w471) -> (number=w476:u32)
        n211 = To Unsigned Byte Integer(number=w476) -> (unsigned 8bit integer=w475:u8)
        n212 = call "SetDioOut.vi"("错误输入（无错误）"=w472, "DioOut"=w475, "DioChanSel"=u8 255, "DevIndex"=w473) -> ("错误输出"=w464:errorcluster, "DevIndex Output"=w465:i32)  [unwired: 6 in]
        n213 = Unbundle(w464) -> ()  [unwired: 3 out]
        n214 = call "GetAiChans.vi"("错误输入（无错误）"=w464, "Num"=u32 1, "ChanSel"=u16 8, "DevIndex"=w465) -> ("错误输出"=w463:errorcluster, "Ai"=w459:sgl[][], "DevIndex Output"=w462:i32)  [unwired: 4 in, 1 out]
        n215 = Index Array(array=w459, index (row)=0, index (col)=0) -> (element=w457:sgl)
        n216 = Divide(x=w457, y=-2.294) -> (x/y=w455:dbl)
        n217 = Bundle(w455, "低负"=w458) -> (w453:cluster{dbl, "低负":sgl})  [unwired: 1 in]
      }
      frame 5 {
        w478 = 0.0
        (unwired) TRUE
        w481 = FALSE
        n218 = call "StartRead.vi"("错误输入（无错误）"=w482, "DevIndex"=w483) -> ("错误输出"=w485:errorcluster, "DevIndex Output"=w486:i32)  [unwired: 8 in]
        n219 = Build Array(w481, w481, w481, w481, w481, w481, w481, w481) -> (w484:bool[])
        n220 = Boolean Array To Number(Boolean array=w484) -> (number=w489:u32)
        n221 = To Unsigned Byte Integer(number=w489) -> (unsigned 8bit integer=w488:u8)
        n222 = call "SetDioOut.vi"("错误输入（无错误）"=w485, "DioOut"=w488, "DioChanSel"=u8 255, "DevIndex"=w486) -> ("错误输出"=w479:errorcluster, "DevIndex Output"=w480:i32)  [unwired: 6 in]
        n223 = Unbundle(w479) -> ()  [unwired: 3 out]
        n224 = Bundle(w478, w478) -> (w477:cluster{dbl, dbl})  [unwired: 1 in]
      }
    }
    "输出气压波形图表" <- w238
    n225 = Unbundle(w238) -> (→"测量值":dbl, "高正"=→"给定值":dbl)
    n226 = case shown="真" "自动破膜" {
      frame False {
      }
      frame True {
        n227 = local read "阻值数组"() -> (w286:dbl[])
        n228 = Index Array(array=w286, index=0 ("索引")) -> (element=w282:dbl)
        n229 = Less?(x=500.0 ("y"), y=w282) -> (x < y?=w284:bool)
        n230 = case shown="真" w284 {
          frame False {
            n231 = local write "自动破膜"(FALSE) -> ()
          }
          frame True {
            n232 = case shown="\"500ms\"" "枚举" {
              tunnel: [200.0 1000.0 500.0] -> w288
              frame "200ms", Default {
              }
              frame "1000ms" {
              }
              frame "500ms" {
              }
            }
            n233 = Tick Count (ms)() -> (millisecond timer value=w290:u32)
            n234 = local read "起始破膜时间"() -> (w293:u32)
            n235 = Subtract(x=w290, y=w293) -> (x-y=w291:u32)
            n236 = Greater?(x=w288, y=w291) -> (0:w292:bool)
            n237 = case shown="假" w292 {
              frame False {
                n238 = flat-sequence {
                  frame #0 {
                    w299 = FALSE
                    n239 = local write "高负开关"(w299) -> ()
                    n240 = local write "低正开关"(w299) -> ()
                    n241 = local write "高正开关"(w299) -> ()
                    n242 = local write "低负开关"(w299) -> ()
                    n243 = local write "大气压"(TRUE) -> ()
                    n244 = local write "case"(5.0) -> ()
                  }
                  frame #1 {
                    n245 = local write "自动破膜"(FALSE ("自动破膜")) -> ()
                  }
                }
              }
              frame True {
                n246 = flat-sequence {
                  frame #0 {
                    w303 = FALSE
                    n247 = local write "高负开关"(TRUE) -> ()
                    n248 = local write "低正开关"(w303) -> ()
                    n249 = local write "高正开关"(w303) -> ()
                    n250 = local write "低负开关"(w303) -> ()
                    n251 = local write "大气压"(w303) -> ()
                    n252 = local write "case"(2.0) -> ()
                  }
                  frame #1 {
                    n253 = local write "高负"(-5.0) -> ()
                  }
                }
              }
            }
          }
        }
      }
    }
  }
  n254 = while {
    tunnel: w111 -> [w499]
    tunnel: [w498] -> w43
    tunnel: w8 -> [w497]
    tunnel: w7 -> [w496]
    stop <- w494 stop-if-true
    # "电流信号循环"
    n255 = Dequeue Element(queue=w497, timeout in ms (-1)=1 ("超时毫秒(-1)"), error in (no error)=w496) -> (error out=w492:errorcluster)  [unwired: 3 out]
    n256 = Unbundle By Name(w492) -> ("status"=w494:bool)
    n257 = flat-sequence {
      tunnel: w499 -> [w520]
      tunnel: [w520] -> w491
      tunnel: [w508] -> w490
      tunnel: [w528] -> w501
      tunnel: [w543] -> w500
      tunnel: w491 -> [w529]
      tunnel: w490 -> [w543]
      tunnel: [w564] -> w505
      tunnel: [w549] -> w504
      tunnel: w501 -> [w544]
      tunnel: w500 -> [w560]
      tunnel: w505 -> [w639]
      tunnel: w504 -> [w640]
      tunnel: w499 -> [w641]
      tunnel: [w638] -> w503
      tunnel: [w630] -> w502
      tunnel: [w683] -> w498
      tunnel: w503 -> [w683]
      tunnel: w502 -> [w681]
      frame #0 {
        n258 = case shown="假" "控制箱刺激ON\n/放大器刺激" {
          tunnel: [0.0 ("data") 5.0 ("data")] -> w517
          frame False {
          }
          frame True {
          }
        }
        n259 = call-poly <vilib>:"DAQmx Create Virtual Channel.vi"("physical channels"=tag "Dev2/ao1") -> ("task out"=w513:refnum<k21>, "error out"=w514:errorcluster)  [unwired: 13 in]
        n260 = call <vilib>:"DAQmx Start Task.vi"("task/channels in"=w513, "error in"=w514) -> ("task out"=w512:refnum<k21>, "error out"=w511:errorcluster)  [unwired: 12 in]
        n261 = call-poly <vilib>:"DAQmx Write.vi"("task/channels in"=w512, "data"=w517, "error in"=w511) -> ("task out"=w510:refnum<k21>, "error out"=w509:errorcluster)  [unwired: 10 in, 1 out]
        n262 = call <vilib>:"DAQmx Stop Task.vi"("task/channels in"=w510, "error in"=w509) -> ("task out"=w516:refnum<k21>, "error out"=w515:errorcluster)  [unwired: 12 in]
        n263 = call <vilib>:"DAQmx Clear Task.vi"("task in"=w516, "error in"=w515) -> ("error out"=w508:errorcluster)  [unwired: 13 in]
      }
      frame #1 {
        n264 = Unbundle By Name(w529) -> ("amplitude"=w535:dbl, "frequency"=w534:dbl, "Fs"=w536:dbl, "Averaging"=w537:i32)
        n265 = Multiply(x=w536, y=w537) -> (x*y=w532:dbl)
        n266 = Multiply(x="钳制电位", y="Holding Voltage") -> (x*y=w525:dbl)
        n267 = Divide(x=w532, y=w534) -> (x/y=w533:dbl)
        n268 = Divide(x=w535, y=2.0) -> (x/y=w539:dbl)
        n269 = Add(x=w525, y=0.5) -> (x+y=w523:dbl)
        "x*y" <- w523
        n270 = Divide(x=w523, y=1000.0) -> (x/y=w540:dbl)
        n271 = Add(x=w540, y=w539) -> (x+y=w530:dbl)
        n272 = Bundle("Fs"=w536, w533) -> (w538:cluster{"Fs":dbl, dbl})  [unwired: 1 in]
        n273 = call <vilib>:"Basic Function Generator.vi"("offset"=w530, "sampling info"=w538, "signal type"=T12."Square Wave", "amplitude"=w539, "frequency"=w534) -> ("signal out"=w528:waveform(dbl))  [unwired: 4 in, 2 out]
      }
      frame #2 {
        w593 = 10178 items=["有限采样"=10178, "连续采样"=10123, "硬件定时单点"=12522] ("sample mode")
        w594 = tag "OnboardClock" ("source")
        w586 = 10178 items=["有限采样"=10178, "连续采样"=10123, "硬件定时单点"=12522] ("sample mode")
        # "必须要有触发"
        # "This version of StimRecord is for the NI DAQ used in conjunction with the MultiClamp 700b"
        # "multiclamp放大器自己参数"
        # "in V"
        # "in nA"
        n274 = case shown="0, 默认" "电压钳/电流钳" {
          tunnel: [50.0 ("y") 2500000000.0 ("y")] -> w561
          tunnel: [2000.0 ("y") 0.1 ("y")] -> w562
          frame 0, Default {
          }
          frame 1 {
          }
        }
        n275 = Multiply(x=w544, y=w561) -> (x*y=w579:waveform(dbl))
        n276 = call-poly <vilib>:"Waveform Duration.vi"("waveform in"=w544) -> ("duration"=w581:dbl)  [unwired: 8 in, 2 out]
        n277 = Unbundle By Name(w579) -> ("Y"=w548:dbl[], "dt"=w578:dbl)
        n278 = for {
          tunnel: [w608] -> w547 mode=indexing
          tunnel: w548 -> [w602] mode=indexing
          w603 = 10.0 ("t")
          w606 = -10.0 ("t")
          n279 = Greater?(x=w606, y=w602) -> (0:w607:bool)
          n280 = Select(t=w606, s=w607, f=w602) -> (s? t:f=w604:dbl)
          n281 = Less?(x=w603, y=w604) -> (x < y?=w605:bool)
          n282 = Select(t=w603, s=w605, f=w604) -> (s? t:f=w608:dbl)
        }
        n283 = Multiply(x=w581, y=2.0) -> (x*y=w582:dbl)
        n284 = Add(x=w582, y=5.0) -> (x+y=w551:dbl)
        n285 = call-poly <vilib>:"DAQmx Create Virtual Channel.vi"("physical channels"=tag "Dev2/ai0", "error in"=w560) -> ("task out"=w585:refnum<k21>, "error out"=w584:errorcluster)  [unwired: 12 in]
        n286 = call-poly <vilib>:"DAQmx Create Virtual Channel.vi"("physical channels"=tag "Dev2/ao0", "error in"=w560) -> ("task out"=w574:refnum<k21>, "error out"=w573:errorcluster)  [unwired: 12 in]
        n287 = Reciprocal(x=w578) -> (1/x=w587:dbl)
        n288 = Array Size(array=w548) -> (size(s)=w601:i32)
        n289 = call-poly <vilib>:"DAQmx Timing.vi"("task/channels in"=w574, "sample mode"=w593, "samples per channel"=w601, "rate"=w587, "source"=w594, "error in"=w573) -> ("task out"=w559:refnum<k21>, "error out"=w557:errorcluster)  [unwired: 8 in]
        n290 = Bundle By Name(cluster=w579, "Y"=w547) -> (w580:waveform(dbl))
        n291 = call-poly <vilib>:"DAQmx Timing.vi"("task/channels in"=w585, "sample mode"=w586, "samples per channel"=w601, "rate"=w587, "source"=w594, "error in"=w584) -> ("task out"=w589:refnum<k21>, "error out"=w590:errorcluster)  [unwired: 8 in]
        n292 = call-poly <vilib>:"DAQmx Trigger.vi"("task/channels in"=w559, "source"=tag "/Dev2/ai/StartTrigger", "error in"=w557) -> ("task out"=w558:refnum<k21>, "error out"=w556:errorcluster)  [unwired: 11 in]
        n293 = call-poly <vilib>:"DAQmx Write.vi"("task/channels in"=w558, "auto start"=FALSE, "data"=w580, "timeout"=w551, "error in"=w556) -> ("task out"=w577:refnum<k21>, "error out"=w598:errorcluster)  [unwired: 8 in, 1 out]
        n294 = property class="DAQmx定时" props=["SampClk.Rate"](reference=w589, error in=w590) -> (reference out=w591:refnum<k21>)  [unwired: 2 out]
        n295 = call <vilib>:"DAQmx Start Task.vi"("task/channels in"=w577, "error in"=w598) -> ("task out"=w595:refnum<k21>, "error out"=w597:errorcluster)  [unwired: 12 in]
        n296 = call <vilib>:"DAQmx Start Task.vi"("task/channels in"=w591, "error in"=w597) -> ("task out"=w569:refnum<k21>, "error out"=w570:errorcluster)  [unwired: 12 in]
        n297 = call-poly <vilib>:"DAQmx Read.vi"("task/channels in"=w569, "number of samples per channel"=w601, "timeout"=w551, "error in"=w570) -> ("task out"=w555:refnum<k21>, "data"=w583:waveform(dbl), "error out"=w553:errorcluster)  [unwired: 9 in]
        n298 = call <vilib>:"DAQmx Is Task Done.vi"("task/channels in"=w595, "error in"=w597) -> ("task out"=w596:refnum<k21>, "error out"=w599:errorcluster)  [unwired: 11 in, 1 out]
        n299 = call <vilib>:"DAQmx Wait Until Done.vi"("task/channels in"=w596, "timeout (sec)"=w551, "error in"=w599) -> ("task out"=w575:refnum<k21>, "error out"=w576:errorcluster)  [unwired: 11 in]
        n300 = call <vilib>:"DAQmx Wait Until Done.vi"("task/channels in"=w555, "timeout (sec)"=w551, "error in"=w553) -> ("task out"=w554:refnum<k21>, "error out"=w552:errorcluster)  [unwired: 11 in]
        n301 = call <vilib>:"DAQmx Stop Task.vi"("task/channels in"=w575, "error in"=w576) -> ("task out"=w572:refnum<k21>, "error out"=w571:errorcluster)  [unwired: 12 in]
        n302 = Multiply(x=w583, y=w562) -> (x*y=w549:waveform(dbl))
        "电流信号波形图" <- w549
        n303 = call <vilib>:"DAQmx Stop Task.vi"("task/channels in"=w554, "error in"=w552) -> ("task out"=w567:refnum<k21>, "error out"=w568:errorcluster)  [unwired: 12 in]
        n304 = call <vilib>:"DAQmx Clear Task.vi"("task in"=w572, "error in"=w571) -> ("error out"=w600:errorcluster)  [unwired: 13 in]
        n305 = call <vilib>:"DAQmx Clear Task.vi"("task in"=w567, "error in"=w568) -> ("error out"=w566:errorcluster)  [unwired: 13 in]
        n306 = Merge Errors(w600, w566) -> (w564:errorcluster)
        n307 = Build Array(w579, w549) -> ()  [unwired: 1 out]
      }
      frame #3 {
        # "数据读取错误"
        # "阻值读取异常处理"
        # "单位换算不明白"
        # "阻值处理"
        # "Convert Volts/pA into MOhms"
        n308 = call "Filter"("error in (no error)"=w639, "Signal"=w640) -> ("error out"=w642:errorcluster, "Filtered Signal"=w634:dynamicdata)  [unwired: 8 in]
        n309 = call "单频测量"("Signals"=w634) -> ("Frequency"=w633:dynamicdata)  [unwired: 9 in, 1 out]
        n310 = Unbundle By Name(w641) -> ("Fs"=w655:dbl, "frequency"=w654:dbl, "Proportion"=w647:dbl)
        n311 = Unbundle By Name(w641) -> ("Averaging"=w653:i32)
        n312 = call "Convert from Dynamic Data"("Dynamic Data Type"=w634) -> ("Array"=w645:dbl[])  [unwired: 3 in]
        n313 = call "从动态数据转换"("Dynamic Data Type"=w633) -> ("Array"=w632:dbl[])  [unwired: 3 in]
        n314 = call-poly <vilib>:"Mean.vi"("X"=w632) -> ("mean"=w629:dbl)  [unwired: 1 out]
        n315 = Divide(x=w655, y=w654) -> (x/y=w658:dbl)
        n316 = Reshape Array(w645, w653, w658) -> (w657:dbl[][])
        n317 = call-poly <vilib>:"Mean.vi"("X"=w645) -> ("mean"=w646:dbl)  [unwired: 1 out]
        n318 = for {
          N: w653 -> [_]
          tunnel: w657 -> [w669] mode=indexing
          tunnel: w642 -> [w676]
          shift-right: [w677] -> w656
          shift-left: dbl[] [] -> [w678]
          tunnel: [w664] -> w652
          tunnel: [w676] -> w638
          tunnel: w647 -> [w668]
          # "不是整个电流的均值"
          # "波形后半段"
          # "波形前半段"
          n319 = Array Size(array=w669) -> (size(s)=w666:i32)
          n320 = Subtract(x=1.0, y=w668) -> (x-y=w671:dbl)
          n321 = Divide(x=w666, y=2) -> (x/y=w673:dbl)
          n322 = Multiply(x=w673, y=w671) -> (x*y=w670:dbl)
          n323 = Split 1D Array(array=w669, index=w673) -> (first subarray=w665:dbl[], second subarray=w674:dbl[])
          n324 = Split 1D Array(array=w665, index=w670) -> (second subarray=w661:dbl[])  [unwired: 1 out]
          n325 = Split 1D Array(array=w674, index=w670) -> (second subarray=w662:dbl[])  [unwired: 1 out]
          n326 = call-poly <vilib>:"Mean.vi"("X"=w661) -> ("mean"=w663:dbl)  [unwired: 1 out]
          n327 = call-poly <vilib>:"Mean.vi"("X"=w662) -> ("mean"=w664:dbl)  [unwired: 1 out]
          n328 = Subtract(x=w663, y=w664) -> (x-y=w667:dbl)
          n329 = Build Array (concatenate)(w678, w667) -> (w677:dbl[])
        }
        "Negative Peak" <- w652
        n330 = Subtract(x=w629, y=sgl 20.0) -> (x-y=w627:dbl)
        n331 = Array Max & Min(array=w645) -> (min value=w644:dbl)  [unwired: 3 out]
        n332 = Absolute Value(x=w627) -> (abs(x)=w626:dbl)
        n333 = Greater?(x=w626, y=0.05) -> (0:w620:bool)
        "！" <- w620
        n334 = Subtract(x=w646, y=w644) -> (x-y=w643:dbl)
        n335 = Unbundle By Name(w641) -> ("amplitude"=w650:dbl)
        n336 = Multiply(x=w650, y=1000000.0) -> (x*y=w637:dbl)
        n337 = Divide(x=w637, y=w643) -> (x/y=→"电阻值":dbl)
        n338 = call-poly <vilib>:"Mean.vi"("X"=w656) -> ("mean"=w651:dbl)  [unwired: 1 out]
        n339 = local read "Resistance(MΩ)"() -> (w623:dbl)
        n340 = Divide(x=w637, y=w651) -> (x/y=w636:dbl)
        n341 = Multiply(x=w636, y=2.0) -> (x*y=w635:dbl)
        n342 = local read "阻值数组"() -> (w631:dbl[])
        n343 = Less?(x=w623, y=100.0) -> (x < y?=w621:bool)
        n344 = And(x=w621, y=w620) -> (x .and. y?=w619:bool)
        n345 = case shown="假" w619 {
          tunnel: w623 -> [_ w660]
          tunnel: w635 -> [w659 _]
          tunnel: [w659 w660] -> w618
          frame False {
          }
          frame True {
          }
        }
        n346 = In Range and Coerce(upper limit=10000.0 ("上限"), x=w618, lower limit=0.0 ("下限")) -> (coerced(x)=w613:dbl)  [unwired: 1 out]
        "阻值波形图表" <- w613
        "Resistance(MΩ)" <- w613
        n347 = Insert Into Array(array=w631, index=0 ("索引"), new element=w613) -> (w630:dbl[])
        n348 = local write "阻值数组"(w630) -> ()
      }
      frame #4 {
        n349 = Array Size(array=w681) -> (size(s)=w680:i32)
        n350 = Greater?(x=w680, y=10) -> (0:w679:bool)
        n351 = case shown="真" w679 {
          tunnel: w681 -> [_ w687]
          frame False {
          }
          frame True {
            n352 = Delete From Array(array=w687, length=1 ("长度"), index=9 ("索引")) -> (array with subset deleted=w684:dbl[])  [unwired: 1 out]
            n353 = local write "阻值数组"(w684) -> ()
          }
        }
      }
    }
    n354 = case shown="真" "入液阻值校准" {
      frame False {
      }
      frame True {
        n355 = flat-sequence {
          frame #0 {
            n356 = local read "Resistance(MΩ)"() -> (→"校准的入液阻值":dbl)
          }
          frame #1 {
            n357 = local write "入液阻值校准"(FALSE) -> ()
          }
        }
      }
    }
  }
  n358 = VISA Close(VISA resource name=w10, error in (no error)=w9) -> ()  [unwired: 1 out]
  n359 = call "IMAQ Create"("Image Name"="二值化") -> ("New Image"=w45:T3)  [unwired: 4 in, 1 out]
  n360 = call "IMAQ Create"("Image Name"="针尖清晰度图像处理") -> ("New Image"=w46:T3)  [unwired: 4 in, 1 out]
  n361 = call "IMAQ Create"("Image Name"="图像检测") -> ("New Image"=w15:T3)  [unwired: 4 in, 1 out]
  n362 = call "IMAQ Create"("Image Name"="mask图像") -> ("New Image"=w13:T3)  [unwired: 4 in, 1 out]
  n363 = while {
    tunnel: w121 -> [w724]
    tunnel: w119 -> [w723]
    tunnel: [w690] -> w114
    shift-right: [w721] -> _
    shift-left: _ -> [w720]
    tunnel: w112 -> [w718]
    tunnel: [w701] -> w110
    tunnel: [w717] -> w109
    tunnel: w108 -> [w716]
    tunnel: [w715] -> w107
    tunnel: w106 -> [w714]
    tunnel: w8 -> [w713]
    tunnel: [w710] -> w104
    shift-right: [w709] -> w103
    shift-left: w7 -> [w708]
    tunnel: w49 -> [w702]
    tunnel: w46 -> [w700]
    tunnel: w45 -> [w699]
    tunnel: w15 -> [w688]
    tunnel: w13 -> [_]
    stop <- "停止" stop-if-true
    (unwired) 2 ("长度")
    # "图像检测"
    # "图像处理循环"
    # "目标坐标"
    n364 = property on="Image" class="ImageControl"() -> ("ROI"=w704:T13)  [unwired: 2 in, 2 out]
    n365 = Unbundle(w704) -> ("Global Rectangle"=w706:i32[])  [unwired: 1 out]
    n366 = Tick Count (ms)() -> (millisecond timer value=w721:u32)
    n367 = call <vilib>:"IMAQdx Grab2.vi"("error in"=w716, "Image In"=w723, "Session In"=w724) -> ("error out"=w715:errorcluster, "Image Out"=w719:T3, "Session Out"=w690:T8)  [unwired: 5 in, 1 out]
    n368 = Array Subset(array=w706, index=0 ("索引")) -> (→"目标坐标":i32[])  [unwired: 1 in]
    n369 = Subtract(x=w721, y=w720) -> (x-y=→"循环时间":u32)
    n370 = call "IMAQ ExtractSingleColorPlane"("error in (no error)"=w714, "Image Dst"=w718, "Image Src"=w719) -> ("error out"=w717:errorcluster, "Image Dst Out"=w701:T3)  [unwired: 7 in]
    n371 = Enqueue Element(queue=w713, element="停止", timeout in ms (-1)=1 ("超时毫秒(-1)"), error in (no error)=w708) -> (queue out=w710:refnum<queue>, error out=w709:errorcluster)  [unwired: 1 out]
    n372 = case shown="真" "针尖模板匹配" {
      tunnel: w702 -> [_ w874]
      tunnel: w701 -> [w834 w838]
      tunnel: [FALSE w873] -> w695
      tunnel: [w833 w841] -> _
      tunnel: [w834 w837] -> w693
      frame False {
        w835 = 0.0 ("x")
        n373 = Bundle("x"=w835, "x"=w835) -> (w833:cluster{"x":dbl, "x":dbl})  [unwired: 1 in]
      }
      frame True {
        w840 = u32 1 items=["Frame", "Fill", "Highlight"] ("Drawing Mode (Frame)")
        w843 = 10.0 ("y")
        w867 = u16 0 items=["All", "Shift Information", "Rotation Information"] ("Learn Mode")
        # "目标和针尖坐标获取"
        # "模板针尖偏移量"
        # "是否匹配到"
        # "模板匹配针尖"
        n374 = call "IMAQ Setup Match Pattern 2"("Minimum Contrast"="Minimum Contrast", "Match Mode"="Match Mode") -> ("Match Pattern Setup Data"=w871:string)  [unwired: 8 in, 1 out]
        n375 = call "IMAQ Setup Learn Pattern 2"("Learn Mode"=w867) -> ("Learn Pattern Setup Data"=w866:string)  [unwired: 9 in, 1 out]
        n376 = call "IMAQ Learn Pattern 2"("Learn Pattern Setup Data"=w866, "Image"=w874) -> ("Template Image Out"=w863:T3)  [unwired: 8 in, 1 out]
        n377 = call "IMAQ Match Pattern 2"("Minimum Match Score"="Minimum Match Score", "Number of Matches Requested"="Number of Matches Requested", "Match Pattern Setup Data"=w871, "Template Image"=w863, "Image"=w838) -> ("Number of Matches"=w864:i32, "Matches"=w860:T7)  [unwired: 4 in, 1 out]
        "Number of Matches" <- w864
        "Matches 2" <- w860
        n378 = Equal?(x=w864, y=0) -> ()  [unwired: 1 out]
        n379 = Index Array(array=w860, index=0 ("索引")) -> (element=w858:T14)
        n380 = Index Array(array=w860, index=0 ("索引")) -> (element=w842:T14)
        n381 = Unbundle(w858) -> ("Score"=w857:sgl)  [unwired: 4 out]
        n382 = Less?(x=w857, y=sgl 800.0) -> (x < y?=w873:bool)
        n383 = Unbundle(w842) -> ("Position"=w841:cluster{"x":sgl, "y":sgl})  [unwired: 4 out]
        n384 = Cluster To Array(cluster=w841) -> (array=→"针尖坐标":sgl[])
        n385 = Unbundle(w841) -> ("x"=w852:sgl, "y"=w855:sgl)
        n386 = Add(x=w852, y=sgl 0.0) -> (x+y=w854:sgl)
        n387 = Subtract(x=w855, y=w843) -> (x-y=w846:dbl)
        n388 = Add(x=w855, y=w843) -> (x+y=w845:dbl)
        n389 = Subtract(x=w854, y=w843) -> (x-y=w844:dbl)
        n390 = Add(x=w854, y=w843) -> (x+y=w847:dbl)
        n391 = To Long Integer(number=w846) -> (32bit integer=w849:i32)
        n392 = To Long Integer(number=w845) -> (32bit integer=w850:i32)
        n393 = To Long Integer(number=w844) -> (32bit integer=w848:i32)
        n394 = To Long Integer(number=w847) -> (32bit integer=w851:i32)
        n395 = Bundle(w848, w849, w851, w850) -> (w839:cluster{i32, i32, i32, i32})  [unwired: 1 in]
        n396 = call "IMAQ Overlay Oval"("Drawing Mode (Frame)"=w840, "Bounding Rectangle"=w839, "Image"=w838) -> ("Image Out"=w837:T3)  [unwired: 7 in, 1 out]
      }
    }
    "Image" <- w693
    "是否匹配到？" <- w695
    n397 = case shown="真" "对比图" {
      tunnel: w693 -> [_ w784]
      frame False {
      }
      frame True {
        n398 = flat-sequence {
          tunnel: w784 -> [w785]
          frame #0 {
            "Image 2" <- w785
          }
          frame #1 {
            n399 = local write "对比图"(FALSE) -> ()
          }
        }
      }
    }
    n400 = local read "针尖细对焦"() -> (w696:bool)
    n401 = local read "针尖粗对焦"() -> (w697:bool)
    n402 = local read "自动扫描"() -> (w692:bool)
    n403 = Or(x=w697, y=w696) -> (x .or. y?=w691:bool)
    n404 = Or(x=w692, y=w691) -> (x .or. y?=w689:bool)
    n405 = case shown="真" w689 {
      tunnel: [0.0 ("Right") w791] -> w698
      tunnel: w693 -> [_ w806]
      tunnel: w700 -> [_ w805]
      tunnel: w699 -> [_ w804]
      frame False {
      }
      frame True {
        n406 = call "IMAQ Threshold"("Range"="Range", "Image Dst"=w804, "Image Src"=w806) -> ("Image Dst Out"=w808:T3)  [unwired: 7 in, 1 out]
        n407 = call "IMAQ LowPass"("Image Src"=w808) -> ("Image Dst Out"=w809:T3)  [unwired: 6 in, 1 out]
        n408 = call "IMAQ Copy"("Image Dst"=w805, "Image Src"=w809) -> ("Image Dst Out"=w816:T3)  [unwired: 4 in, 1 out]
        n409 = call "IMAQ RemoveParticle"("Number of Erosion"="Number of Erosion", "Image Src"=w816) -> ("Image Dst Out"=w810:T3)  [unwired: 8 in, 1 out]
        n410 = call "IMAQ Morphology"("Operation"="Operation", "Image Src"=w810) -> ("Image Dst Out"=w813:T3)  [unwired: 8 in, 1 out]
        n411 = call "IMAQ Convex Hull"("Image Src"=w813) -> ("Image Dst Out"=w814:T3)  [unwired: 9 in, 1 out]
        n412 = call "IMAQ FillHole"("Image Src"=w814) -> ("Image Dst Out"=w811:T3)  [unwired: 5 in, 1 out]
        n413 = call "IMAQ Clear Overlay"("Image"=w811) -> ("Image Out"=w803:T3)  [unwired: 9 in, 1 out]
        "二值化" <- w803
        n414 = call "IMAQ Particle Analysis Report"("Image"=w803) -> ("Particle Reports (Pixels)"=w807:T6)  [unwired: 5 in, 5 out]
        "Particle Reports (Pixels)" <- w807
        n415 = call "IMAQ Particle Analysis"("Pixel Measurements"="Pixel Measurements", "Image"=w803) -> ("Particle Measurements (Pixels)"=w796:dbl[][])  [unwired: 4 in, 5 out]
        "Particle Measurements (Pixels)" <- w796
        n416 = Array Max & Min(array=w796) -> (max value=w801:dbl)  [unwired: 3 out]
        "startY" <- w801
        n417 = while {
          tunnel: w807 -> [w818]
          shift-right: [w827] -> w791
          shift-left: _ -> [w822]
          i -> [w820]
          stop <- w824 stop-if-true
          n418 = Equal?(x=w820, y=0) -> (x = y?=w821:bool)
          n419 = case shown="真" w821 {
            tunnel: w822 -> [w831 _]
            tunnel: [w831 0] -> w819
            frame False {
            }
            frame True {
            }
          }
          n420 = Index Array(array=w818, index=w820) -> (element=w829:T15)
          n421 = Unbundle(w829) -> ("Bounding Rect"=w830:T16)  [unwired: 5 out]
          n422 = Unbundle(w830) -> ("Right"=w825:dbl)  [unwired: 3 out]
          n423 = Equal?(x=w825, y=0.0) -> (x = y?=w824:bool)
          n424 = Greater?(x=w819, y=w825) -> (0:w828:bool)
          n425 = Select(t=w819, s=w828, f=w825) -> (s? t:f=w827:dbl)
        }
        "Right" <- w791
        n426 = Greater?(x=w791, y=200.0) -> (0:w793:bool)
        n427 = Greater?(x=w801, y=200.0) -> (0:w800:bool)
        n428 = Less?(x=w801, y=1800.0) -> (x < y?=w799:bool)
        n429 = Less?(x=w791, y=1800.0) -> (x < y?=w794:bool)
        n430 = And(x=w800, y=w799) -> (x .and. y?=w790:bool)
        n431 = And(x=w793, y=w794) -> (x .and. y?=w789:bool)
        n432 = And(x=w790, y=w789) -> (x .and. y?=w788:bool)
        n433 = local write "手动暂停"(w788) -> ()
      }
    }
    "清晰度评价函数" <- w698
    n434 = case shown="真" {
      selector: _ -> [_ _]
      tunnel: w688 -> [_ w725]
      frame False {
      }
      frame True {
        n435 = stacked-sequence {
          tunnel: w725 -> [_ _ _ w744]
          frame #0 {
            n436 = local read "Image"() -> (w727:T3)
            n437 = call-poly "IMAQ Write File 2"("File Path"=path "C:/Users/Administrator/Desktop/1.bmp", "Image"=w727) -> ()  [unwired: 8 in, 2 out]
          }
          frame #1 {
            n438 = Wait (ms)(milliseconds to wait=u32 1000 ("等待时间（毫秒）")) -> ()  [unwired: 1 out]
          }
          frame #2 {
            w734 = path "D:/韩宇/程序/自动膜片钳系统/test.txt" ("文件路径（使用对话框）")
            n439 = Get File Size(file=w734) -> (size (in bytes)=w735:i64)  [unwired: 1 in, 2 out]
            n440 = Open/Create/Replace File(file path (use dialog)=w734) -> (refnum out=w732:refnum<file>)  [unwired: 5 in, 2 out]
            n441 = Negate(x=w735) -> (-x=w736:i64)
            n442 = Set File Position(offset (in bytes) (0)=w736, refnum=w732, from (0:start)=enum16{"start", "end", "current"}."end" ("自（0:起始）")) -> (refnum out=w733:refnum<file>, error out=w738:errorcluster)  [unwired: 1 in]
            n443 = Read from Text File(file (use dialog)=w733, count=-1 ("计数"), error in=w738) -> (refnum out=w739:refnum<file>, text=w741:string[], error out=w740:errorcluster)  [unwired: 1 in, 1 out]
            n444 = Reverse 1D Array(array=w741) -> (reversed array=w730:string[])
            n445 = Close File(refnum=w739, error in=w740) -> ()  [unwired: 2 out]
            n446 = Index Array(array=w730, index=0 ("索引")) -> (element=→"元素":string)
          }
          frame #3 {
            # "tcp通信"
            n447 = local read "Image"() -> (w743:T3)
            n448 = call "IMAQ Extract 2"("Optional Rectangle"=i32[] [], "Image Dst"=w744, "Image Src"=w743) -> ("Image Dst Out"=w747:T3)  [unwired: 7 in, 1 out]
            n449 = TCP Open Connection(address="10.134.224.218" ("名称"), remote port or service name=u16 8888 ("远程端口或服务名称")) -> (connection ID=w746:refnum<k5>)  [unwired: 3 in, 1 out]
            n450 = call "IMAQ ImageToArray"("Image"=w747) -> ("Image Pixels (U8)"=w750:u8[][])  [unwired: 3 in, 4 out]
            n451 = for {
              tunnel: w750 -> [w765] mode=indexing
              tunnel: [w764] -> w751 mode=indexing
              n452 = for {
                tunnel: w765 -> [w766] mode=indexing
                tunnel: [w767] -> w764 mode=indexing
                n453 = Less?(x=w766, y=u8 10) -> (x < y?=w768:bool)
                n454 = case shown="假" w768 {
                  tunnel: [w770 w782] -> w767
                  tunnel: w766 -> [w771 w783]
                  frame False {
                    n455 = Less?(x=w771, y=u8 100) -> (x < y?=w772:bool)
                    n456 = case shown="真" w772 {
                      tunnel: w771 -> [w775 w777]
                      tunnel: [w774 w776] -> w770
                      frame False {
                        n457 = Number To Decimal String(number=w775) -> (decimal integer string=w774:string)  [unwired: 1 in]
                      }
                      frame True {
                        n458 = Number To Decimal String(number=w777) -> (decimal integer string=w779:string)  [unwired: 1 in]
                        n459 = Concatenate Strings("0" ("字符串"), w779) -> (w776:string)
                      }
                    }
                  }
                  frame True {
                    n460 = Number To Decimal String(number=w783) -> (decimal integer string=w781:string)  [unwired: 1 in]
                    n461 = Concatenate Strings("00" ("字符串"), w781) -> (w782:string)
                  }
                }
              }
            }
            n462 = Concatenate Strings(w751) -> (w749:string)
            n463 = flat-sequence {
              tunnel: w749 -> [w756]
              tunnel: [w757] -> w752
              tunnel: w746 -> [w755]
              tunnel: [w763] -> w748
              tunnel: w752 -> [w760]
              frame #0 {
                (unwired) "hello" ("数据输入")
                n464 = TCP Write(connection ID=w755, data in=w756) -> (connection ID out=w757:refnum<k5>, bytes written=→"写入的字节 2":i32)  [unwired: 2 in, 1 out]
              }
              frame #1 {
                n465 = TCP Read(connection ID=w760, bytes to read=7 ("读取的字节"), 7:"模式（标准） 2") -> (connection ID out=w763:refnum<k5>, data out=→"数据输出 2":string)  [unwired: 2 in, 1 out]
              }
            }
            n466 = TCP Close Connection(connection ID=w748) -> ()  [unwired: 2 in, 2 out]
          }
        }
      }
    }
  }
  n467 = Get Date/Time String(date format (0)=enum16{"short", "long", "abbreviated"}."long" ("日期格式(0)"), want seconds? (F)=TRUE ("需要秒？(F)")) -> (date string=w39:string, time string=w24:string)  [unwired: 1 in]
  n468 = String Subset(string=w24, offset (0)=6 ("偏移量(0)")) -> (substring=w22:string)  [unwired: 1 in]
  n469 = String Subset(string=w24, offset (0)=3 ("偏移量(0)"), length (rest)=2 ("长度（剩余）")) -> (substring=w34:string)
  n470 = String Subset(string=w24, length (rest)=2 ("长度（剩余）")) -> (substring=w36:string)  [unwired: 1 in]
  n471 = Concatenate Strings(w36, "时" ("字符串"), w34, "分" ("字符串"), w22, "秒" ("字符串")) -> (w35:string)
  n472 = Concatenate Strings(w39, w35) -> (w18:string)
  n473 = Build Path(base path=path "E:/膜片/实验/数据" ("文件路径（使用对话框）"), name or relative path=w18) -> (appended path=w32:path)
  n474 = call "SetDA.vi"("错误输入（无错误）"=w11, "DevIndex"=w12) -> ("错误输出"=w75:errorcluster, "DevIndex Output"=w76:i32)  [unwired: 8 in]
  n475 = Create Folder(path (use dialog)=w32) -> (created path=w27:path)  [unwired: 2 in, 2 out]
  n476 = Build Path(base path=w27, name or relative path="data.txt" ("字符串")) -> (appended path=w29:path)
  n477 = call "SetDA.vi"("错误输入（无错误）"=w75, "DAVolt"=0.0, "DANum"=u8 1, "DevIndex"=w76) -> ("错误输出"=w74:errorcluster, "DevIndex Output"=w73:i32)  [unwired: 6 in]
  n478 = Open/Create/Replace File(file path (use dialog)=w29, operation (0:open)=T9."open or create" ("操作(0:open)")) -> (refnum out=w28:refnum<file>)  [unwired: 4 in, 2 out]
  n479 = while {
    tunnel: w6 -> [w875]
    tunnel: w7 -> [w897]
    tunnel: [w888] -> w41
    tunnel: w8 -> [w896]
    tunnel: w28 -> [w886]
    tunnel: w27 -> [w885]
    tunnel: [w883] -> w26
    tunnel: w5 -> [w881]
    tunnel: [w876] -> w1
    i -> [w884]
    stop <- w898 stop-if-true
    # "Mp285A控制循环"
    n480 = Dequeue Element(queue=w896, timeout in ms (-1)=1 ("超时毫秒(-1)"), error in (no error)=w897) -> (error out=w899:errorcluster)  [unwired: 3 out]
    n481 = Unbundle By Name(w899) -> ("status"=w898:bool)
    n482 = flat-sequence {
      tunnel: [w1065] -> w895
      tunnel: w875 -> [w1065]
      tunnel: w895 -> [w1068]
      tunnel: [w1069] -> w894
      tunnel: w894 -> [w1152]
      tunnel: [w1151] -> w893
      frame #0 {
        n483 = event shown="[1] 超时" {
          selector: _ -> [_ _]
          dyn-events: _ -> [_ _]
          timeout: 1 -> [_ _]
          event "自动接触": Value Change {
            n484 = event-data() -> ()  [unwired: 1 in, 6 out]
            "自动接触初始" <- 0
          }
          event Timeout {
            n485 = event-data() -> ()  [unwired: 1 in, 3 out]
          }
        }
      }
      frame #1 {
        n486 = local read "Right"() -> (w1070:dbl)
        n487 = case shown="真" "针尖粗对焦" {
          tunnel: w1070 -> [_ w1073]
          tunnel: w1068 -> [w1072 w1074]
          tunnel: [w1072 w1075] -> w1069
          frame False {
          }
          frame True {
            # "爬山算法"
            # "聚焦有问题"
            n488 = flat-sequence {
              tunnel: w1073 -> [w1135]
              tunnel: [w1149] -> w1081
              tunnel: [w1148] -> w1079
              tunnel: [w1147] -> w1080
              frame #0 {
                n489 = case shown="1" "自动对焦状态机" {
                  tunnel: w1135 -> [w1136 w1143]
                  frame 0, Default {
                    n490 = flat-sequence {
                      tunnel: w1136 -> [w1140]
                      frame #0 {
                        n491 = Array Size(array="聚焦值数组") -> (size(s)=w1139:i32)
                        n492 = Delete From Array(array="聚焦值数组", length=w1139) -> (array with subset deleted=w1138:dbl[])  [unwired: 1 in, 1 out]
                        n493 = local write "聚焦值数组"(w1138) -> ()
                      }
                      frame #1 {
                        # "第一次赋值"
                        "调焦值2" <- w1140
                        "调焦值3" <- w1140
                        "调焦值4" <- w1140
                        "对焦变量" <- 1
                      }
                      frame #2 {
                        n494 = local write "自动对焦状态机"(1) -> ()
                      }
                    }
                  }
                  frame 1 {
                    n495 = flat-sequence {
                      tunnel: w1143 -> [w1146]
                      frame #0 {
                        n496 = local read "调焦值3"() -> (w1144:dbl)
                        n497 = local write "调焦值4"(w1144) -> ()
                      }
                      frame #1 {
                        n498 = local read "调焦值2"() -> (w1145:dbl)
                        n499 = local write "调焦值3"(w1145) -> ()
                      }
                      frame #2 {
                        n500 = local write "调焦值2"(w1146) -> ()
                      }
                    }
                  }
                }
              }
              frame #1 {
                n501 = local read "调焦值2"() -> (w1149:dbl)
                n502 = local read "调焦值3"() -> (w1148:dbl)
                n503 = local read "调焦值4"() -> (w1147:dbl)
              }
            }
            n504 = local read "聚焦值数组"() -> (w1077:dbl[])
            n505 = Insert Into Array(array=w1077, new element=w1073) -> (w1078:dbl[])  [unwired: 1 in]
            n506 = local write "聚焦值数组"(w1078) -> ()
            n507 = Greater?(x=w1079, y=w1080) -> (0:w1087:bool)
            n508 = Greater?(x=w1081, y=w1079) -> (0:w1084:bool)
            n509 = Boolean To (0,1)(Boolean=w1084) -> (0, 1=w1083:i16)
            n510 = Boolean To (0,1)(Boolean=w1087) -> (0, 1=w1082:i16)
            n511 = Multiply(x=i16 10, y=w1083) -> (x*y=w1085:i16)
            n512 = Add(x=w1085, y=w1082) -> (x+y=w1076:i16)
            "x+y 2" <- w1076
            n513 = case shown="1" w1076 {
              tunnel: w1074 -> [w1089 w1098 w1113 w1117]
              tunnel: [w1088 w1097 w1109 w1116] -> w1075
              frame 10 {
                # "4继续向上运动"
                n514 = flat-sequence {
                  tunnel: [w1095] -> w1088
                  tunnel: w1089 -> [w1094]
                  frame #0 {
                    n515 = local read "对焦变量"() -> (w1092:dbl)
                    n516 = Multiply(x=5.0 ("Z 2"), y=w1092) -> (x*y=w1090:dbl)
                    n517 = call "285_RelMove.vi"("VISA资源名称"=w1094, "Z 2"=w1090, "Y 2"=0.0, "X 2"=0.0) -> ("VISA resource name out 2"=w1095:refnum<visa-resource-name>)  [unwired: 2 in, 5 out]
                  }
                }
              }
              frame 0 {
                # "2向回运动"
                n518 = flat-sequence {
                  tunnel: w1098 -> [w1108]
                  tunnel: [w1107] -> w1097
                  frame #0 {
                    n519 = local read "对焦变量"() -> (w1101:dbl)
                    n520 = Multiply(x=-1.0 ("y"), y=w1101) -> (x*y=w1099:dbl)
                    n521 = local write "对焦变量"(w1099) -> ()
                  }
                  frame #1 {
                    n522 = local read "对焦变量"() -> (w1104:dbl)
                    n523 = Multiply(x=5.0, y=w1104) -> (x*y=w1102:dbl)
                    n524 = call "285_RelMove.vi"("VISA资源名称"=w1108, "Z 2"=w1102, "Y 2"=0.0, "X 2"=0.0) -> ("VISA resource name out 2"=w1107:refnum<visa-resource-name>)  [unwired: 2 in, 5 out]
                  }
                }
              }
              frame 11, Default {
                # "1往上运动"
                n525 = local read "对焦变量"() -> (w1111:dbl)
                n526 = Multiply(x=5.0 ("Z 2"), y=w1111) -> (x*y=w1110:dbl)
                n527 = call "285_RelMove.vi"("VISA资源名称"=w1113, "Z 2"=w1110, "Y 2"=0.0, "X 2"=0.0) -> ("VISA resource name out 2"=w1109:refnum<visa-resource-name>)  [unwired: 2 in, 5 out]
              }
              frame 1 {
                # "3最大值停止运动"
                n528 = local read "聚焦值数组"() -> (w1123:dbl[])
                n529 = Array Max & Min(array=w1123) -> (max value=w1122:dbl)  [unwired: 3 out]
                n530 = local read "Right"() -> (w1119:dbl)
                n531 = Subtract(x=w1122, y=5.0) -> (x-y=w1120:dbl)
                n532 = Greater?(x=w1119, y=w1120) -> (0:w1118:bool)
                n533 = case shown="假" w1118 {
                  tunnel: w1117 -> [w1128 w1132]
                  tunnel: [w1124 w1132] -> w1116
                  frame False {
                    n534 = local read "对焦变量"() -> (w1125:dbl)
                    n535 = Multiply(x=5.0 ("Z 2"), y=w1125) -> (x*y=w1127:dbl)
                    n536 = call "285_RelMove.vi"("VISA资源名称"=w1128, "Z 2"=w1127, "Y 2"=0.0, "X 2"=0.0) -> ("VISA resource name out 2"=w1124:refnum<visa-resource-name>)  [unwired: 2 in, 5 out]
                  }
                  frame True {
                    n537 = local write "自动对焦状态机"(0) -> ()
                    n538 = local write "针尖粗对焦"(FALSE ("针尖粗对焦")) -> ()
                  }
                }
              }
            }
          }
        }
      }
      frame #2 {
        n539 = local read "是否匹配到？"() -> (w1150:bool)
        n540 = And(x=w1150, y="针尖细对焦") -> (x .and. y?=w1153:bool)
        n541 = case shown="假" w1153 {
          tunnel: w1152 -> [w1156 w1163]
          tunnel: [w1156 w1162] -> w1151
          frame False {
            n542 = local write "针尖细对焦"(FALSE ("针尖细对焦")) -> ()
          }
          frame True {
            n543 = local read "对焦变量"() -> (w1159:dbl)
            n544 = Multiply(x=2.0, y=w1159) -> (x*y=w1157:dbl)
            n545 = call "285_RelMove.vi"("VISA资源名称"=w1163, "Z 2"=w1157, "Y 2"=0.0, "X 2"=0.0) -> ("VISA resource name out 2"=w1162:refnum<visa-resource-name>)  [unwired: 2 in, 5 out]
          }
        }
      }
    }
    n546 = case shown="真" "自动移至工作位置" {
      tunnel: w881 -> [w946 w955]
      tunnel: w875 -> [w947 w952]
      tunnel: [w947 w949] -> w877
      tunnel: [w946 w948] -> w876
      frame False {
      }
      frame True {
        n547 = flat-sequence {
          tunnel: w955 -> [w958]
          tunnel: [w956] -> w954
          tunnel: w954 -> [w965]
          tunnel: [w965] -> w953
          tunnel: w953 -> [w977]
          tunnel: w952 -> [w976]
          tunnel: [w977] -> w951
          tunnel: [w966] -> w950
          tunnel: [w980] -> w949
          tunnel: [w981] -> w948
          tunnel: w951 -> [w981]
          tunnel: w950 -> [w980]
          frame #0 {
            n548 = call "285_GetPos.vi"("VISA资源名称"=w958) -> ("Y"=→"Y":dbl, "X"=→"X":dbl, "VISA资源名称输出"=w956:refnum<visa-resource-name>)  [unwired: 5 in, 3 out]
          }
          frame #1 {
            n549 = local read "Z轴坐标"() -> (w961:string)
            n550 = Decimal String To Number(string=w961) -> (number=w960:i32)  [unwired: 2 in, 1 out]
            n551 = To Double Precision Float(number=w960) -> (double precision float=w962:dbl)
            n552 = Divide(x=w962, y=10.0) -> (x/y=→"Z":dbl)
          }
          frame #2 {
            # "标定"
            n553 = local read "Z"() -> (w973:dbl)
            n554 = local read "Y"() -> (w974:dbl)
            n555 = local read "X"() -> (w975:dbl)
            n556 = Add(x=w973, y=-25108.0) -> (x+y=w967:dbl)
            n557 = Add(x=w974, y=4961.0) -> (x+y=w968:dbl)
            n558 = Add(x=w975, y=-20810.0) -> (x+y=w969:dbl)
            n559 = call "285_Move.vi"("VISA resource name out"=w976, "Abso_Z"=w967, "Abso_Y"=w968, "Abso_X"=w969) -> ("VISA resource name out 2"=w966:refnum<visa-resource-name>)  [unwired: 4 in, 3 out]
          }
          frame #3 {
            n560 = local write "自动移至工作位置"(FALSE) -> ()
            n561 = local write "自动扫描"(TRUE) -> ()
          }
        }
      }
    }
    n562 = case shown="真" "自动扫描" {
      tunnel: w877 -> [_ w910]
      frame False {
      }
      frame True {
        n563 = case shown="2" "自动扫描状态机" {
          tunnel: w910 -> [w911 w918 _]
          frame 0, Default {
            # "初始状态"
            n564 = flat-sequence {
              tunnel: w911 -> [w912]
              frame #0 {
                n565 = call "285_RelMove.vi"("VISA资源名称"=w912, "Z 2"=0.0, "Y 2"=50.0 ("X 2"), "X 2"=0.0 ("Y 2")) -> ()  [unwired: 2 in, 6 out]
                "扫描变量" <- -1.0 ("扫描变量")
              }
              frame #1 {
                n566 = local write "自动扫描状态机"(u16 1) -> ()
              }
            }
          }
          frame 1 {
            n567 = case shown="真" "手动暂停" {
              tunnel: w918 -> [w923 _]
              frame False {
                n568 = flat-sequence {
                  tunnel: [w929] -> w922
                  tunnel: w923 -> [w930]
                  tunnel: w922 -> [w932]
                  tunnel: [w932] -> w921
                  tunnel: w921 -> [w937]
                  tunnel: [w933] -> w920
                  tunnel: [w941] -> _
                  tunnel: w920 -> [w941]
                  frame #0 {
                    n569 = local read "扫描变量"() -> (w926:dbl)
                    n570 = Multiply(x=500.0 ("X 2"), y=w926) -> (x*y=w924:dbl)
                    n571 = call "285_RelMove.vi"("VISA资源名称"=w930, "Z 2"=0.0, "Y 2"=w924, "X 2"=0.0 ("Y 2")) -> ("VISA resource name out 2"=w929:refnum<visa-resource-name>)  [unwired: 2 in, 5 out]
                  }
                  frame #1 {
                    n572 = Wait (ms)(milliseconds to wait=u32 100 ("等待时间（毫秒）")) -> ()  [unwired: 1 out]
                  }
                  frame #2 {
                    n573 = call "285_RelMove.vi"("VISA资源名称"=w937, "Z 2"=0.0, "Y 2"=0.0 ("X 2"), "X 2"=-20.0 ("Y 2")) -> ("VISA resource name out 2"=w933:refnum<visa-resource-name>)  [unwired: 2 in, 5 out]
                  }
                  frame #3 {
                    n574 = local read "扫描变量"() -> (w940:dbl)
                    n575 = Multiply(x=w940, y=-1.0) -> (x*y=w938:dbl)
                    n576 = local write "扫描变量"(w938) -> ()
                  }
                }
              }
              frame True {
                n577 = flat-sequence {
                  frame #0 {
                    n578 = local write "自动扫描状态机"(2) -> ()
                  }
                  frame #1 {
                  }
                }
              }
            }
          }
          frame 2 {
            n579 = flat-sequence {
              frame #0 {
                n580 = local write "自动扫描状态机"(0) -> ()
              }
              frame #1 {
                w945 = FALSE
                n581 = local write "自动扫描"(w945) -> ()
                n582 = local write "手动暂停"(w945) -> ()
                n583 = local write "针尖粗对焦"(TRUE) -> ()
              }
            }
          }
        }
      }
    }
    n584 = case shown="真" "手动换物镜" {
      tunnel: w877 -> [_ w902]
      frame False {
      }
      frame True {
        n585 = flat-sequence {
          tunnel: w902 -> [w908]
          frame #0 {
            n586 = One Button Dialog(message="请手动更换40倍显微镜" ("消息")) -> ()  [unwired: 1 in, 1 out]
          }
          frame #1 {
            n587 = call "285_RelMove.vi"("VISA资源名称"=w908, "Z 2"=10.0, "Y 2"=0.0, "X 2"=0.0) -> ()  [unwired: 2 in, 6 out]
            n588 = local write "手动换物镜"(FALSE) -> ()
          }
        }
      }
    }
    n589 = local read "针尖坐标"() -> (w891:sgl[])
    n590 = local read "目标坐标"() -> (w892:i32[])
    n591 = case shown="真" "针尖自动移动" {
      tunnel: w893 -> [w1019 w1042]
      tunnel: [w1019 w1029] -> w882
      tunnel: w892 -> [_ w1031]
      tunnel: w891 -> [_ w1024]
      frame False {
      }
      frame True {
        # "模板针尖偏移量"
        # "PID控制针尖移动"
        # "可以直接用pid模块"
        n592 = Index Array(array=w1024, index=1 ("索引")) -> (element=w1021:sgl)
        n593 = Index Array(array=w1024, index=0 ("索引")) -> (element=w1020:sgl)
        n594 = Index Array(array=w1031, index=1 ("索引")) -> (element=w1040:i32)
        n595 = Index Array(array=w1031, index=0 ("索引")) -> (element=w1041:i32)
        n596 = Subtract(x=w1040, y=w1021) -> (x-y=w1036:sgl)
        n597 = Bundle("x"=w1021, w1040) -> ()  [unwired: 1 in, 1 out]
        n598 = Add(x=sgl 0.0 ("y"), y=w1020) -> (x+y=w1025:sgl)
        n599 = Subtract(x=w1041, y=w1025) -> (x-y=w1037:sgl)
        n600 = call-poly <vilib>:"PID.vi"("PID gains"="PID gains", "process variable"=w1025, "setpoint"=w1041) -> ("output"=w1027:dbl)  [unwired: 7 in, 1 out]
        n601 = call-poly <vilib>:"PID.vi"("PID gains"="PID gains 2", "process variable"=w1021, "setpoint"=w1040) -> ("output"=w1028:dbl)  [unwired: 7 in, 1 out]
        n602 = Bundle("x"=w1020, w1041) -> ()  [unwired: 1 in, 1 out]
        n603 = Square(x=w1037) -> (x^2=w1035:sgl)
        n604 = Square(x=w1036) -> (x^2=w1034:sgl)
        n605 = Add(x=w1035, y=w1034) -> (x+y=w1030:sgl)
        n606 = Greater?(x=w1030, y=15.0) -> (0:w1043:bool)
        n607 = case shown="假" w1043 {
          tunnel: w1042 -> [w1047 w1051]
          tunnel: [w1047 w1050] -> w1029
          tunnel: w1027 -> [_ w1049]
          tunnel: w1028 -> [_ w1048]
          frame False {
            n608 = local write "针尖自动移动"(FALSE) -> ()
            n609 = One Button Dialog(message="针尖已移动到目标位置" ("消息")) -> ()  [unwired: 1 in, 1 out]
          }
          frame True {
            # "阈值范围需要调整，太大针尖检测不出来，太小程序会出现bug'"
            n610 = flat-sequence {
              tunnel: w1051 -> [w1058]
              tunnel: [w1057] -> w1050
              tunnel: w1049 -> [w1053]
              tunnel: w1048 -> [w1052]
              frame #0 {
                # "x位置p负号原因是设备转换后的"
                n611 = To Byte Integer(number=w1052) -> (8bit integer=w1056:i8)
                n612 = To Byte Integer(number=w1053) -> (8bit integer=w1055:i8)
                n613 = In Range and Coerce(upper limit=2.0 ("上限"), x=w1056, lower limit=-2.0 ("上限")) -> (coerced(x)=w1061:dbl)  [unwired: 1 out]
                n614 = In Range and Coerce(upper limit=2.0 ("上限"), x=w1055, lower limit=-2.0 ("上限")) -> (coerced(x)=w1054:dbl)  [unwired: 1 out]
                n615 = call "285_RelMove.vi"("VISA资源名称"=w1058, "Z 2"=0.0 ("Z"), "Y 2"=w1061, "X 2"=w1054) -> ("VISA resource name out 2"=w1057:refnum<visa-resource-name>)  [unwired: 2 in, 5 out]
              }
            }
          }
        }
      }
    }
    n616 = case shown="真" "自动接触" {
      tunnel: w882 -> [w1164 w1178]
      tunnel: [w1164 w1174] -> w889
      frame False {
      }
      frame True {
        # "阈值"
        n617 = local read "校准的入液阻值"() -> (w1173:dbl)
        n618 = local read "阻值数组"() -> (w1184:dbl[])
        n619 = local read "自动接触初始"() -> (w1166:i32)
        n620 = Index Array(array=w1184, index=0 ("索引")) -> (element=w1177:dbl)
        n621 = Index Array(array=w1184, index=1 ("索引")) -> (element=w1182:dbl)
        n622 = Index Array(array=w1184, index=2 ("索引")) -> (element=w1181:dbl)
        n623 = Multiply(x=1.01, y=w1173) -> (x*y=w1171:dbl)
        n624 = Greater Or Equal?(x=w1177, y=w1182) -> (x >= y?=w1180:bool)
        n625 = Greater Or Equal?(x=w1182, y=w1181) -> (x >= y?=w1179:bool)
        n626 = Greater?(x=w1177, y=w1171) -> (0:w1176:bool)
        n627 = And(x=w1180, y=w1179) -> (x .and. y?=w1175:bool)
        n628 = And(x=w1176, y=w1175) -> (x .and. y?=w1167:bool)
        n629 = Boolean To (0,1)(Boolean=w1167) -> (0, 1=w1168:i16)
        n630 = Multiply(x=i16 10, y=w1168) -> (x*y=w1169:i16)
        n631 = Add(x=w1169, y=w1166) -> (x+y=w1165:i32)
        n632 = case shown="10" w1165 {
          tunnel: w1178 -> [w1188 w1208 w1218]
          tunnel: [w1187 w1209 w1218] -> w1174
          frame 10 {
            # "向下运动"
            n633 = case shown="真" "下降/向右 2" {
              tunnel: [0.0 ("X 2") w1200] -> w1191
              tunnel: [w1195 0.0 ("X 2")] -> w1190
              tunnel: [0.0 ("Y 2") 0.0 ("Y 2")] -> w1189
              frame False {
                n634 = local read "下降步伐/um 2"() -> (w1196:dbl)
                n635 = Multiply(x=w1196, y=-10.0) -> (x*y=w1195:dbl)
              }
              frame True {
                n636 = Multiply(x="下降步伐/um 2", y=-10.0) -> (x*y=w1200:dbl)
              }
            }
            n637 = local write "自动接触初始"(1) -> ()
            n638 = call "285_RelMove.vi"("VISA资源名称"=w1188, "Z 2"=w1191, "Y 2"=w1189, "X 2"=w1190) -> ("VISA resource name out 2"=w1187:refnum<visa-resource-name>)  [unwired: 2 in, 5 out]
          }
          frame 0, 1, Default {
            # "向下运动"
            n639 = case shown="真" "下降/向右" {
              tunnel: [0.0 ("X 2") "下降步伐/um"] -> w1206
              tunnel: [w1212 0.0 ("X 2")] -> w1205
              tunnel: [0.0 ("Y 2") 0.0 ("Y 2")] -> w1204
              frame False {
                n640 = local read "下降步伐/um"() -> (w1212:dbl)
              }
              frame True {
              }
            }
            n641 = call "285_RelMove.vi"("VISA资源名称"=w1208, "Z 2"=w1206, "Y 2"=w1204, "X 2"=w1205) -> ("VISA resource name out 2"=w1209:refnum<visa-resource-name>)  [unwired: 2 in, 5 out]
          }
          frame 11 {
            n642 = local write "自动接触"(FALSE) -> ()
            n643 = local write "自动封接"(TRUE) -> ()
            n644 = One Button Dialog(message="电极已接触细胞" ("消息")) -> ()  [unwired: 1 in, 1 out]
          }
        }
      }
    }
    n645 = case shown="真" "保存数据" {
      tunnel: w889 -> [w1002 w1018]
      tunnel: [w993 w1018] -> w888
      tunnel: w886 -> [w995 w1017]
      tunnel: w885 -> [w991 _]
      tunnel: [w994 w1017] -> w883
      tunnel: w884 -> [w989 _]
      frame True {
        w985 = "\t"
        n646 = local read "Resistance(MΩ)"() -> (w992:dbl)
        n647 = call "285_GetPos.vi"("VISA资源名称"=w1002) -> ("Z"=w997:dbl, "Y"=w999:dbl, "X"=w1001:dbl, "VISA资源名称输出"=w993:refnum<visa-resource-name>)  [unwired: 5 in, 2 out]
        n648 = Quotient & Remainder(x=w989, y=100) -> (x-y*floor(x/y)=w987:i32)  [unwired: 1 out]
        n649 = Get Date/Time String(want seconds? (F)=TRUE ("需要秒？(F)")) -> (time string=w983:string)  [unwired: 2 in, 1 out]
        n650 = Number To Fractional String(number=w999) -> (F-format string=w998:string)  [unwired: 3 in]
        n651 = Number To Decimal String(number=w989) -> (decimal integer string=w990:string)  [unwired: 1 in]
        n652 = Number To Fractional String(number=w1001) -> (F-format string=w1000:string)  [unwired: 3 in]
        n653 = Number To Fractional String(number=w997) -> (F-format string=w996:string)  [unwired: 3 in]
        n654 = Number To Fractional String(number=w992) -> (F-format string=w1008:string)  [unwired: 3 in]
        n655 = Equal?(x=w987, y=0) -> (x = y?=w982:bool)
        n656 = case shown="真" w982 {
          tunnel: w991 -> [_ w1012]
          tunnel: w990 -> [_ w1010]
          frame False {
          }
          frame True {
            n657 = Concatenate Strings("图像" ("字符串"), w1010, ".bmp" ("字符串")) -> (w1014:string)
            n658 = local read "Image"() -> (w1011:T3)
            n659 = Build Path(base path=w1012, name or relative path=w1014) -> (appended path=w1016:path)
            n660 = call-poly "IMAQ Write File 2"("File Path"=w1016, "Image"=w1011) -> ()  [unwired: 8 in, 2 out]
          }
        }
        n661 = Concatenate Strings(w983, w985, w990, w985, w985, "X轴：" ("字符串"), w1000, w985, "Y轴：" ("字符串"), w998, w985, "Z轴：" ("字符串"), w996, w985, "阻值：" ("字符串"), w1008, "\n") -> (w1003:string)
        n662 = Write to Text File(file (use dialog)=w995, text=w1003) -> (refnum out=w994:refnum<file>)  [unwired: 2 in, 2 out]
      }
      frame False {
      }
    }
  }
  n663 = Build Array(w64, w64, w64, w64, w64, w64, w64, w64) -> (w62:bool[])
  n664 = call "SetDA.vi"("错误输入（无错误）"=w74, "DAVolt"=0.0, "DANum"=u8 2, "DevIndex"=w73) -> ("错误输出"=w71:errorcluster, "DevIndex Output"=w72:i32)  [unwired: 6 in]
  n665 = Boolean Array To Number(Boolean array=w62) -> (number=w63:u32)
  n666 = call "SetDA.vi"("错误输入（无错误）"=w71, "DAVolt"=0.0, "DANum"=u8 3, "DevIndex"=w72) -> ("错误输出"=w58:errorcluster, "DevIndex Output"=w59:i32)  [unwired: 6 in]
  n667 = To Unsigned Byte Integer(number=w63) -> (unsigned 8bit integer=w61:u8)
  n668 = call "SetDioOut.vi"("错误输入（无错误）"=w58, "DioOut"=w61, "DioChanSel"=u8 255, "DevIndex"=w59) -> ("错误输出"=w57:errorcluster, "DevIndex Output"=w56:i32)  [unwired: 6 in]
  n669 = call "StopRead.vi"("错误输入（无错误）"=w57, "DevIndex"=w56) -> ("错误输出"=w82:errorcluster, "DevIndex Output"=w83:i32)  [unwired: 8 in]
  n670 = call "IMAQ Dispose"("Image"=w110, "error in (no error)"=w109) -> ("error out"=w115:errorcluster)  [unwired: 4 in]
  n671 = call <vilib>:"IMAQdx Close Camera.vi"("error in"=w107, "Session In"=w114) -> ("error out"=w116:errorcluster)  [unwired: 9 in]
  n672 = call "SetSoftTrig.vi"("错误输入（无错误）"=w82, "Trig"=u8 0, "DevIndex"=w83) -> ("错误输出"=w81:errorcluster, "DevIndex Output"=w79:i32)  [unwired: 7 in]
  n673 = Release Queue(queue=w104, error in (no error)=w103) -> (error out=w54:errorcluster)  [unwired: 1 in, 2 out]
  n674 = call "ClearTrigger.vi"("错误输入（无错误）"=w81, "DevIndex"=w79) -> ("错误输出"=w80:errorcluster, "DevIndex Output"=w78:i32)  [unwired: 8 in]
  n675 = Merge Errors(w115, w116, w54) -> (→"错误输出":errorcluster)
  n676 = call "ClearBufs.vi"("错误输入（无错误）"=w80, "DevIndex"=w78) -> ("错误输出"=w84:errorcluster, "DevIndex Output"=w85:i32)  [unwired: 8 in]
  n677 = call "CloseDevice.vi"("错误输入（无错误）"=w84, "DevIndex"=w85) -> ("错误输出"=w42:errorcluster)  [unwired: 8 in, 1 out]
  n678 = Merge Errors(w43, w42) -> (→"错误输出 3":errorcluster)
  n679 = call "285_Update.vi"("VISA资源名称"=w1) -> ("VISA资源名称 2"=w2:refnum<visa-resource-name>)  [unwired: 9 in, 1 out]
  n680 = Close File(refnum=w26) -> ()  [unwired: 1 in, 2 out]
  n681 = call "285_Update.vi"("VISA资源名称"=w41) -> ("VISA资源名称 2"=w44:refnum<visa-resource-name>)  [unwired: 9 in, 1 out]
  n682 = VISA Close(VISA resource name=w2) -> ()  [unwired: 1 in, 1 out]
  n683 = VISA Close(VISA resource name=w44) -> ()  [unwired: 1 in, 1 out]
